vi "Navigation_start_cases_florida_rev3_joystick_cleaned.vi"() -> ()   [LabVIEW 2015]
uses:
  <vilib>/myRIO/Instrument Drivers/Onboard IO/PWM/typedefs/PWM Reference.ctl
  <vilib>/myRIO/Common/Instrument Driver Framework/Utilities/typedefs/myRIO Generic Hardware Reference.ctl
  <vilib>/myRIO/Common/Instrument Driver Framework/Utilities/typedefs/Hardware Version Enum.ctl
  <vilib>/myRIO/Common/Instrument Driver Framework/Utilities/typedefs/myRIO v1.0 Reference.ctl
  <vilib>/myRIO/Common/Instrument Driver Framework/Utilities/typedefs/Generic FPGA Reference.ctl
  <vilib>/myRIO/Common/Instrument Driver Framework/myRIO v1.0/PWM/typedefs/PWM Channels Enum.ctl
  <vilib>/myRIO/Instrument Drivers/Onboard IO/PWM/typedefs/PWM Configuration.ctl
  <vilib>/userdefined/High Color/nirio_resource_hc.ctl
  <vilib>/myRIO/Common/Instrument Driver Framework/myRIO v1.0/PWM/vis/myRIO v1.1 Open PWM.vi
  <vilib>/myRIO/Common/Instrument Driver Framework/Utilities/vis/Validate Channels.vi
  <vilib>/myRIO/Common/Instrument Driver Framework/myRIO v1.0/PWM/vis/myRIO v1.0 Reserve PWM.vi
  <vilib>/myRIO/Common/Instrument Driver Framework/myRIO v1.0/PWM/vis/myRIO v1.0 Build MUX Configuration PWM.vi
  <vilib>/myRIO/Common/Instrument Driver Framework/myRIO v1.0/Resource Manager/vis/myRIO v1.0 Reserve Channel List.vi
  <vilib>/myRIO/Common/Instrument Driver Framework/myRIO v1.0/Resource Manager/vis/myRIO v1.0 Create Configuration List.vi
  <vilib>/myRIO/Common/Instrument Driver Framework/myRIO v1.0/Resource Manager/vis/myRIO v1.0 Reserve Channel.vi
  <vilib>/myRIO/Common/Instrument Driver Framework/myRIO v1.0/Resource Manager/vis/myRIO v1.0 Unreserve Channel.vi
  <vilib>/myRIO/Common/Instrument Driver Framework/myRIO v1.0/Resource Manager/vis/myRIO v1.0 Build Mutex Name.vi
  <vilib>/FPGAPlugInAG/myRIO-1900/niLvFpga_Open_myRIO-1900.vi
  <vilib>/rvi/interface/common/dynamic/niFpgaDynamicAddResources.vi
  <vilib>/myRIO/Common/Instrument Driver Framework/Utilities/vis/FPGA Ref Manager.vi
  <vilib>/Utility/error.llb/Error Cluster From Error Code.vi
  <vilib>/myRIO/Common/Instrument Driver Framework/Utilities/vis/Ref Counter.vi
  <vilib>/rvi/errors/niLvFpgaAdjustHostInterfaceError.vi
  <vilib>/Utility/VariantDataType/GetNumericInfo.vi
  <vilib>/myRIO/Common/Instrument Driver Framework/myRIO v1.0/myRIO v1.1 Open.vi
  <vilib>/myRIO/Common/Instrument Driver Framework/Utilities/vis/IO Manager.vi
  <vilib>/myRIO/Common/Instrument Driver Framework/Utilities/vis/Configuration Manager.vi
  <vilib>/myRIO/Common/Instrument Driver Framework/myRIO v1.0/Resource Manager/vis/myRIO v1.0 Configure IO.vi
  <vilib>/myRIO/Common/Instrument Driver Framework/myRIO v1.0/myRIO v1.0 Close.vi
  <vilib>/myRIO/Common/Instrument Driver Framework/myRIO v1.0/PWM/vis/myRIO v1.0 Write PWM.vi
  <vilib>/addons/control/pid/pid.llb/PID (DBL).vi
  <vilib>/rvi/interface/nirviOpenFPGA/nirviOpenFPGA.xnode
  FPGA Bitfiles/NavigationProjec_FPGATarget2_FPGAMainNavigati_PWPHW8gwDxI.lvbitx
  <vilib>/rvi/interface/nirviReadWriteControl/nirviReadWriteControl.xnode
  <vilib>/myRIO/Instrument Drivers/Onboard IO/PWM/vis/myRIO PWM Open.xnode
  <vilib>/myRIO/Instrument Drivers/Onboard IO/PWM/PWM.lvlib
  <vilib>/myRIO/Instrument Drivers/Utilities/Utilities.lvlib
  NiFpgaLv.dll
  <vilib>/rvi/interface/Simulation/niFpgaSimulationCallBeginRW.vi
  <vilib>/addons/control/pid/NI_PID_pid.lvlib
panel:
  in  "left setpoint 7":dbl=0.06
  in  "right setpoint 7":dbl=0.06
  in  "left setpoint 6":dbl=0.06
  in  "right setpoint 6":dbl=0.06
  in  "right setpoint 5":dbl=0.1
  in  "left setpoint 5":dbl=0.06 format="%#_13g"
  in  "right setpoint 4":dbl=0.06
  in  "left setpoint 4":dbl=0.1
  in  "left setpoint 3":dbl=0.05
  in  "right setpoint 3":dbl=0.1
  in  "left setpoint 2":dbl=0.08 format="%#_13g"
  in  "right setpoint 2":dbl=0.05
  in  "y goal lower limit return":dbl=1.5
  in  "y goal upper limit return":dbl=3.5
  in  "y goal upper limit mine":dbl=9.0
  in  "y goal lower limit mine":dbl=5.0
  in  "dump y":dbl=2.5 format="%#_13g"
  out "angle goal":dbl
  out "y goal":dbl
  in  "dump x":dbl=2.0
  in  "timer control":u32=750
  in  "dumping complete":bool
  in  "digging complete?":bool
  out "start condition":dbl format="%#_13g"
  out "xstart_return":dbl
  out "start x 2":dbl=1.0
  out "goal reached 2":bool=TRUE
  out "percent away from x goal 2":dbl
  in  "x goal":dbl=9.0
  out "goal reached":bool=TRUE
  out "percent away from x goal":dbl
  in  "t backward 6":u32=3000
  in  "Tab Control":enum32{"start a", "start b"}(tab)
  in  "?":T1(tab)=enum."back arc 4 4"
  in  "right 0":dbl=-0.05
  in  "left 0":dbl=-0.05
  in  "t backward 7":u32=3000
  in  "left 1":dbl=0.1
  in  "right 1":dbl=0.05
  in  "right 2":dbl=0.05
  in  "left 2":dbl=0.1
  in  "t backward":u32=3000
  in  "t forward":u32=750
  in  "t forward once":u32=3000
  in  "right once":dbl=0.05
  in  "left once":dbl=0.1
  in  "left 7":dbl=0.1
  in  "right 7":dbl=0.05
  in  "t forward 2":u32=750
  in  "left 6":dbl=0.1
  in  "right 6":dbl=0.05
  in  "t backward 2":u32=3000
  in  "left once 2":dbl=0.1
  in  "right once 2":dbl=0.05
  in  "t forward once 2":u32=3000
  in  "left 12":dbl=0.1
  in  "right 12":dbl=0.05
  in  "left 11":dbl=0.1
  in  "right 11":dbl=0.05
  in  "left 10":dbl=0.1
  in  "right 10":dbl=0.05
  in  "forward":u32=5000
  in  "timeforward":u32=750
  in  "timeback":u32=750
  in  "Tab Control 3":T2(tab)
  in  "left 15":dbl=-0.05
  in  "right 15":dbl=-0.05
  in  "t backward 8":u32=3000
  in  "left 5":dbl=0.1
  in  "right 5":dbl=0.05
  in  "left 4":dbl=0.1
  in  "right 4":dbl=0.05
  in  "left 3":dbl=0.1
  in  "right 3":dbl=0.05
  in  "forward 6":u32=750
  in  "backward 6":u32=750
  in  "onetime 6":u32=5000
  in  "t forward once 5":u32=3000
  in  "right once 5":dbl=0.05
  in  "left once 5":dbl=0.1
  in  "left 16":dbl=0.1
  in  "right 16":dbl=0.05
  in  "t backward 5":u32=3000
  in  "left 17":dbl=0.1
  in  "right 17":dbl=0.05
  in  "t forward 5":u32=750
  in  "start condition":dbl=8.0
  out "big red button":i16
  out "y1ahead":dbl=0.09107784569025501
  out "angle error":dbl=1.4898186625859124
  out "y desired":dbl=-7.9788842668421
  out "slope desired":dbl=12.322079916445226
  out "orientation theta desired":dbl=1.4898186625859124
  out "current angle":dbl
  out "current y":dbl
  out "current x":dbl
  out "mining angle":dbl
  out "mining y":dbl
  out "mining x":dbl
  out "mining location":dbl=-1.0
  out "distance to goal":dbl=-5.348200626633382
  out "loc_y":dbl=1.4807790517807007
  out "loc_x":dbl=3.651799373366618
  out "loc_theta":dbl
  in  "motor killswitch":bool
  in  "state":dbl
  in  "Encoder Reset":bool
  out "scale":dbl
  out "reset x y 2":dbl=1.0
  out "stop motors":dbl
  out "encoder stop switch":dbl=1.0
  out "left wheels actual pwm":dbl=0.5
  out "right wheels actual pwm":dbl=0.5
  out "desired pwm right":dbl=0.5
  out "desired pwm left":dbl=0.5
  out "left setpoint":dbl
  out "right setpoint":dbl
  in  "PID Settings":enum32{"Right PID PWM", "Left PID PWM"}(tab)
  in  "output range right":cluster{"output high":dbl, "output low":dbl}={"output high"=0.15, "output low"=-0.15} {"output low" format="%.6f"; "output high" format="%.5f"}
  in  "PID gains right":T3={"proportional gain (Kc)"=0.002, "integral time (Ti, min)"=7e-07, "derivative time (Td, min)"=0.0} {"derivative time (Td, min)" format="%.8f"; "integral time (Ti, min)" format="%.8f"; "proportional gain (Kc)" format="%.8f"}
  out "dt out (s) right":dbl=0.003000000142492354 format="%.3f"
  out "PID feedback Right":dbl
  out "Elapsed Time (s) Right":dbl=3.140906810760498 caption="Elapsed Time (s)"
  in  "pid reset right":bool
  in  "output range left":cluster{"output high":dbl, "output low":dbl}={"output high"=0.15, "output low"=-0.15} {"output low" format="%.6f"; "output high" format="%.5f"}
  in  "PID gains left":T3={"proportional gain (Kc)"=0.002, "integral time (Ti, min)"=7e-07, "derivative time (Td, min)"=0.0} {"derivative time (Td, min)" format="%.8f"; "integral time (Ti, min)" format="%.8f"; "proportional gain (Kc)" format="%.8f"}
  out "dt out (s) left":dbl=0.003000000142492354 format="%.3f"
  out "PID feedback Left":dbl
  out "Elapsed Time (s) Left":dbl=3.15102481842041 caption="Elapsed Time (s)"
  in  "pid reset left":bool
  out "start angle":dbl
  out "start x":dbl=3.5057763724032824
  out "start y":dbl=1.4807790517807007
  in  "stuff that i dont want to mess with right now":T4(tab)
  out "RM Linear Velocity (rot/s)":dbl
  out "RR Rot Velocity (rot/s)":dbl
  out "LR Rot Velocity (rot/s)":dbl
  out "LM Rot Velocity (rot/s)":dbl
  out "LF Rot Velocity (rot/s)":dbl
  out "RF Linear Velocity (rot/s)":dbl
  out "Tick Count(mSec) 2":u32=223952 caption="Tick Count(mSec)"
  out "y traveled 2":dbl
  out "x traveled 2":dbl
  out "y position 2":dbl=1.4807790517807007
  out "x position 2":dbl=3.5057763724032824
  out "y dot 2":dbl
  out "distance traveled 2":dbl
  out "psi dot 2":dbl
  out "x dot 2":dbl
  out ".not. x? 2":bool
  out ".not. x? 3":bool
  out "avg ENC.B":dbl
  out "avg ENC.A":dbl
  out "ENC.B_c.CNTR":i32
  out "ENC.B_b.CNTR":i32
  out "ENC.B_a.CNTR":i32
  out "ENC.A_c.CNTR":i32
  out "ENC.A_b.CNTR":i32
  out "ENC.A_a.CNTR":i32
  out "stage set point parameters":T5(tab)=enum."mining location -1"
  in  "x straight 1 end":dbl=2.0
  in  "ypstart straight 1":dbl
  in  "ystart":dbl=1.0
  in  "yend straight 1":dbl=2.0
  in  "ypend straight 1":dbl
  out "a":dbl=1.7573967372023482
  out "b":dbl=-14.513750148940964
  out "c":dbl=36.96623974933568
  out "d":dbl=-23.9366528005263
  out "x turn end":dbl=7.0
  out "x straight 2 end":dbl=10.0
  in  "mining y 1":dbl=2.0
  in  "mining angle 1":dbl
  in  "mining x 1":dbl=20.0
  in  "mining angle -1":dbl
  in  "mining y -1":dbl=7.0
  in  "mining x -1":dbl=20.0
  # "go up in y"
  # "go down in y"
  # "go straight"
  # "Position Information"
  # "straight arc back straight arc arc"
  # "move cases along"
  # "end state 0\ngo to state 1"
  # "end state 1\ngo to state 2"
  # "end state 2\ngo to state 3"
  # "end state 3\ngo to state 4"
  # "end state 4\ngo to state 0"
  # "same thing, redundant \nbut can be changed to \nsomething useful later"
  # "this must be true to \ninitialize the routine"
  # "go through the 3\n movement cases"
  # "go through the 3\n movement cases"
  # "same as the start a arc arc"
  # "Stop Flags \n1=go \n0=stop"
  # "PWM Setpoint"
  # "Initial condtions"
  # "Encoder Values"
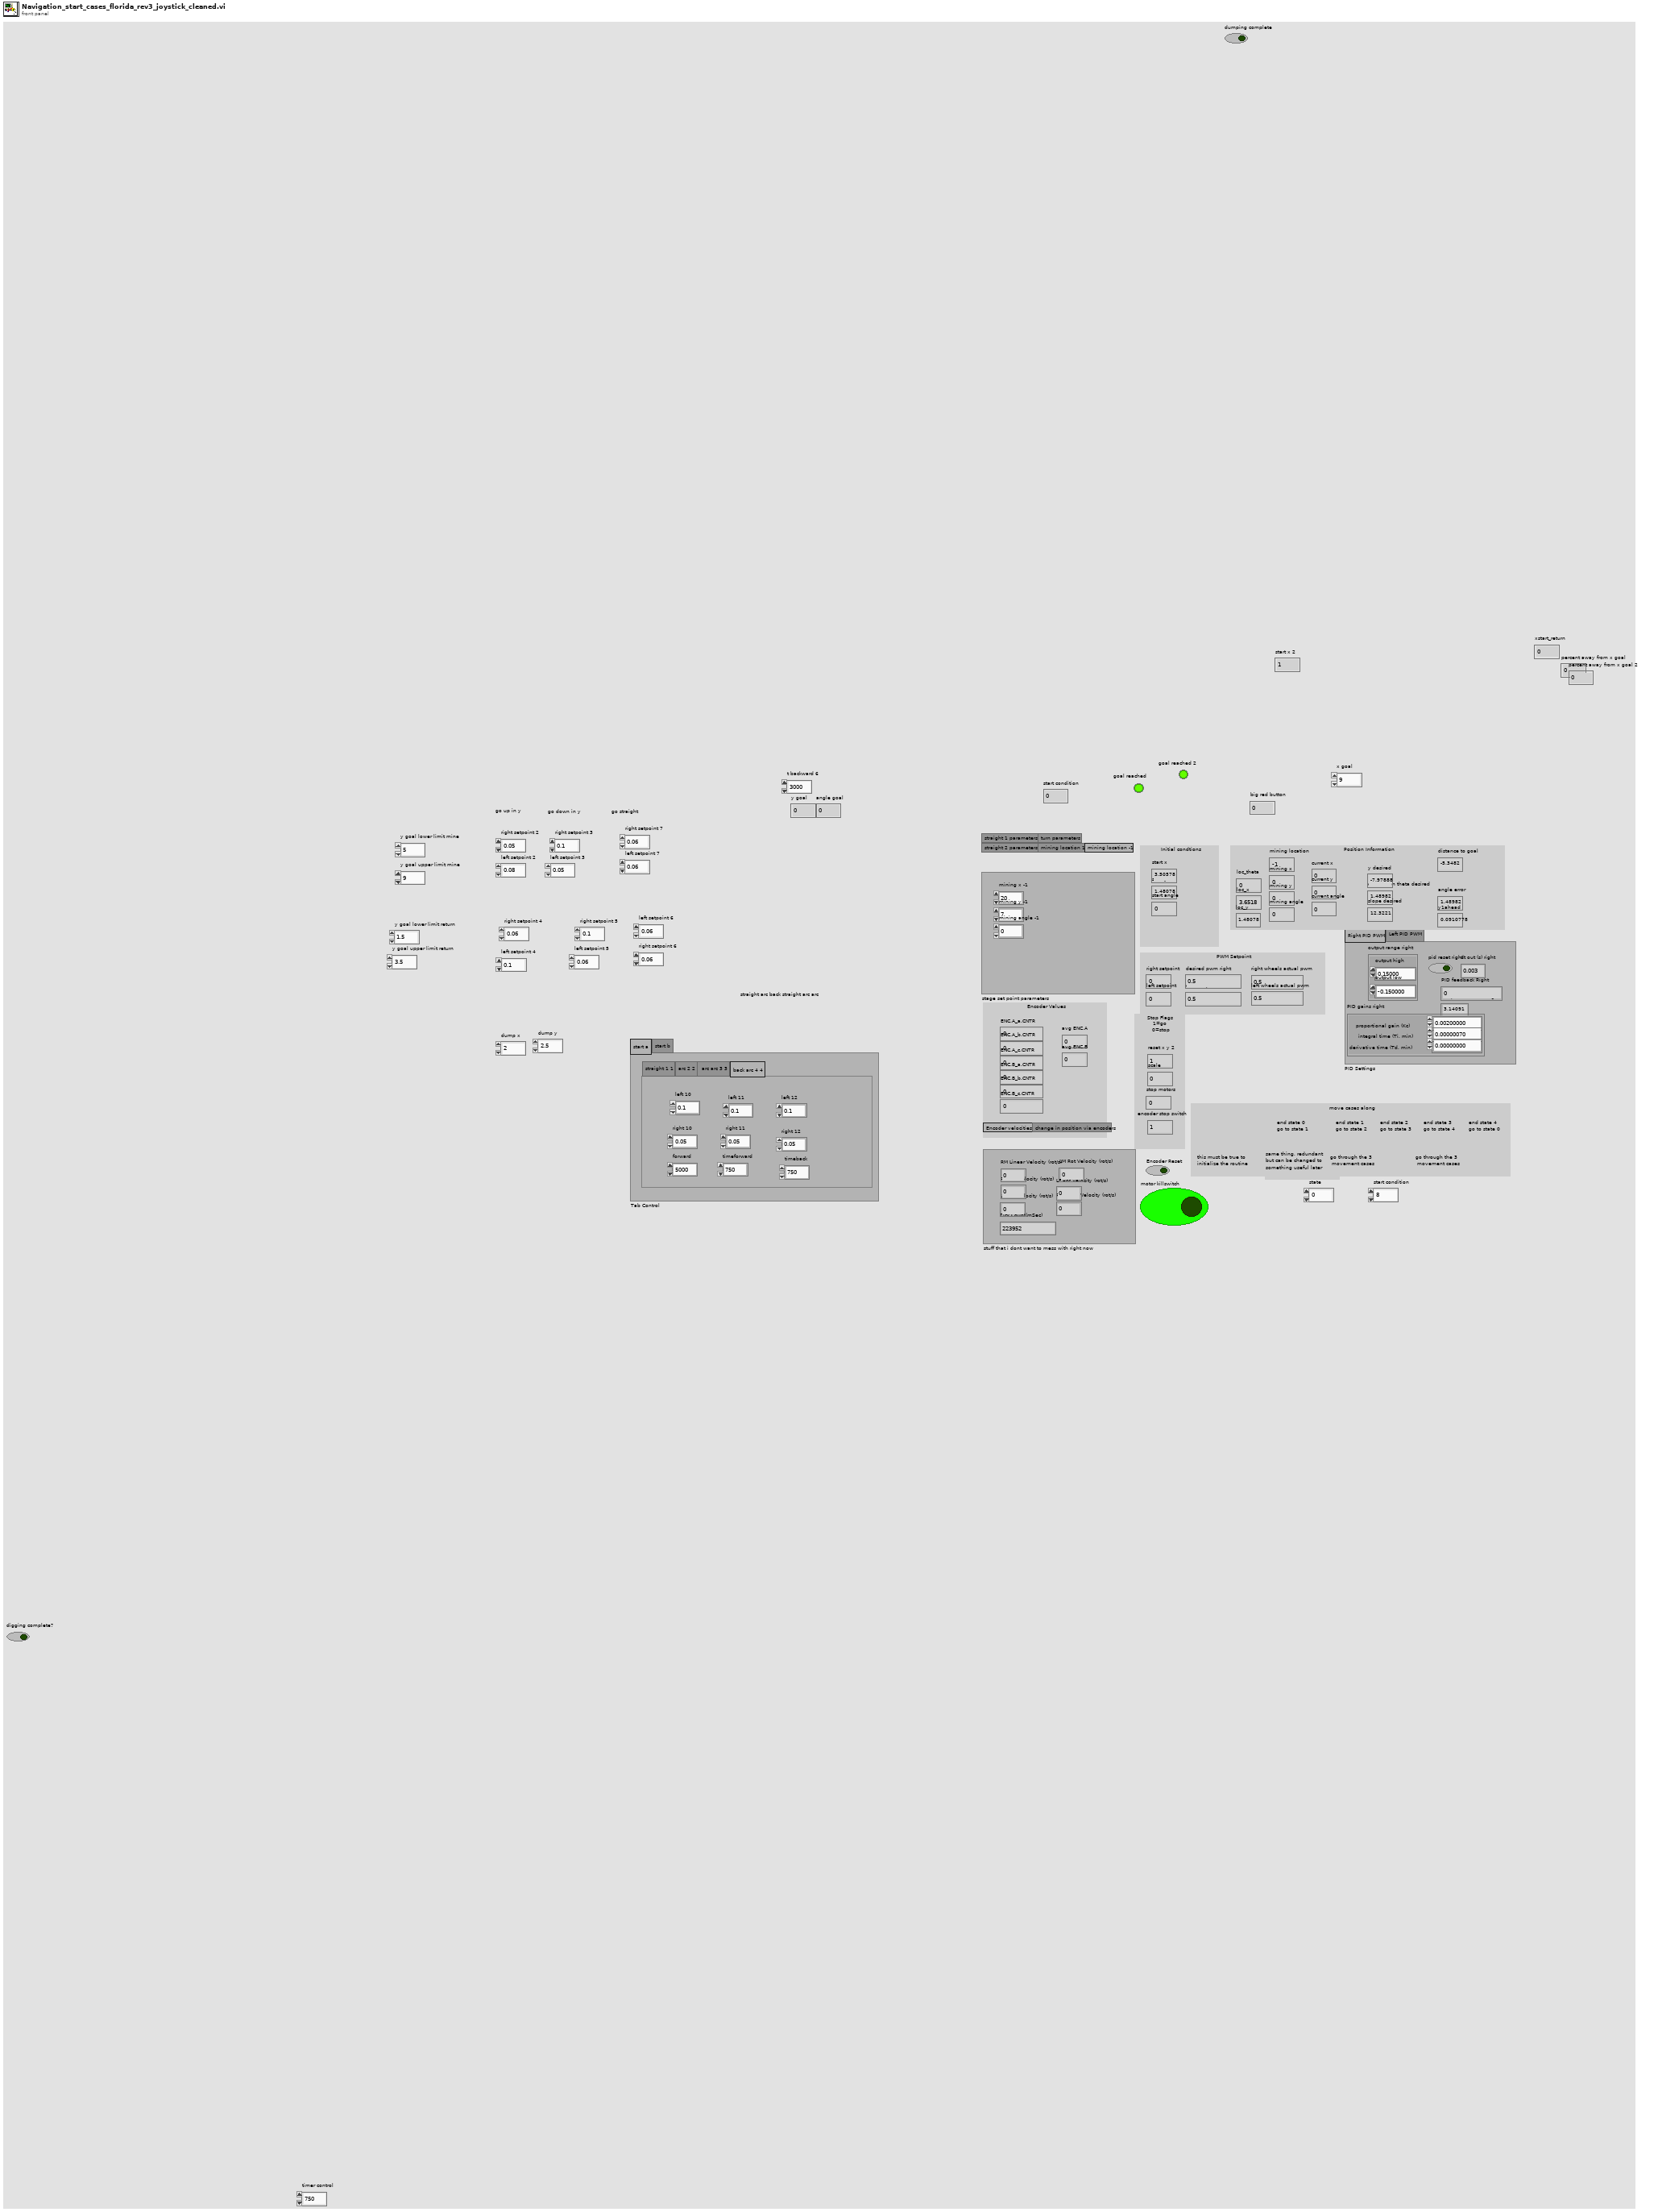
[diagram p1: front panel]
types:
  T1 = enum32{"straight 1 1", "arc 2 2", "arc arc 3 3 ", "back arc 4 4"}
  T2 = enum32{"straight 1 5", "arc 2 6", "arc arc 3", "back arc 4 7"}
  T3 = cluster{"proportional gain (Kc)":dbl, "integral time (Ti, min)":dbl, "derivative time (Td, min)":dbl}
  T4 = enum32{"Encoder velocities", "change in position via encoders"}
  T5 = enum32{"straight 1 parameters", "turn parameters", "straight 2 parameters", "mining location 1", "mining location -1"}
  T6 = typedef "nirio_resource_hc.ctl" = tag
  T7 = typedef "Hardware Version Enum.ctl" = enum16{"Unknown", "myRIO-1900", "myRIO-1950", "roboRIO"}
  T8 = typedef "PWM.lvlib/PWM Reference.ctl" = cluster{"myRIO Reference":T9, "PWM Channels Enum":T12, "PWM Configuration":T13}
  T9 = typedef "myRIO Generic Hardware Reference.ctl" = cluster{"myRIO Model":T7, "myRIO Hardware Reference":T10}
  T10 = typedef "myRIO v1.0 Reference.ctl" = cluster{"Generic FPGA Reference":T11, "Allow multiple opens":bool}
  T11 = typedef "Generic FPGA Reference.ctl" = refnum<k20>
  T12 = typedef "PWM Channels Enum.ctl" = enum16{"Not Connected", "C/PWM0", "C/PWM1", "A/PWM0", "A/PWM1", "A/PWM2", "B/PWM0", "B/PWM1", "B/PWM2", "PWM/PWM0", "PWM/PWM1", "PWM/PWM2", "PWM/PWM3", "PWM/PWM4", "PWM/PWM5", "PWM/PWM6", "PWM/PWM7", "PWM/PWM8", "PWM/PWM9"}
  T13 = typedef "PWM.lvlib/PWM Configuration.ctl" = cluster{"Frequency":dbl, "Duty Cycle":dbl}
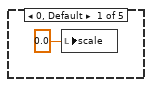
[diagram p3: hidden frame]
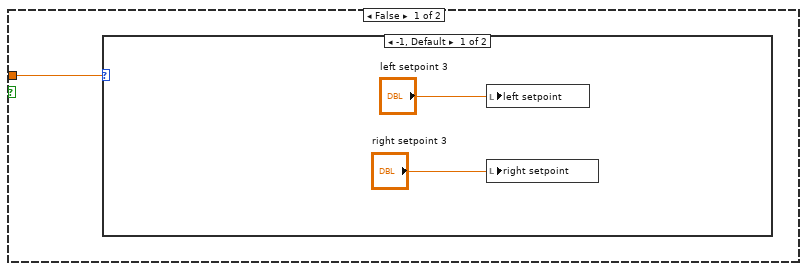
[diagram p4: hidden frame]
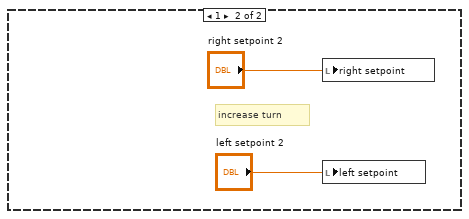
[diagram p5: hidden frame]
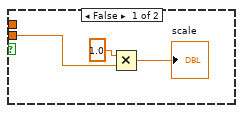
[diagram p6: hidden frame]
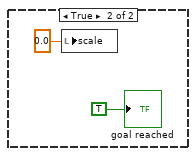
[diagram p7: hidden frame]
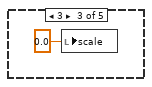
[diagram p8: hidden frame]
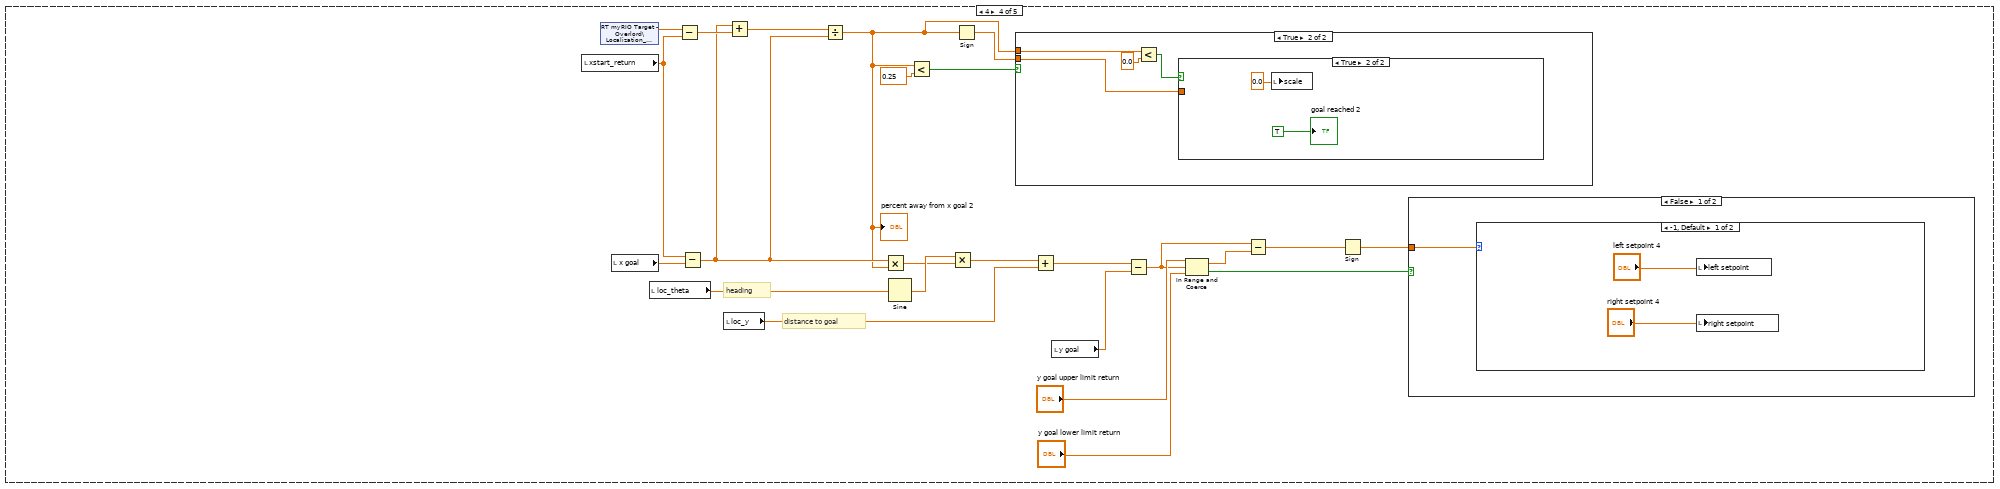
[diagram p9: hidden frame]
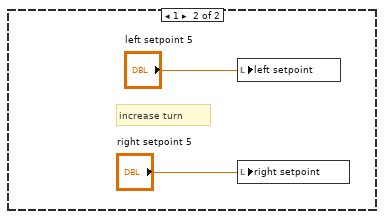
[diagram p10: hidden frame]
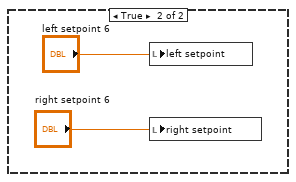
[diagram p11: hidden frame]
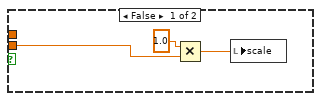
[diagram p12: hidden frame]
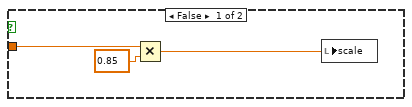
[diagram p13: hidden frame]
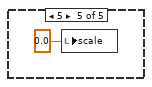
[diagram p14: hidden frame]
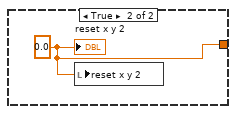
[diagram p15: hidden frame]
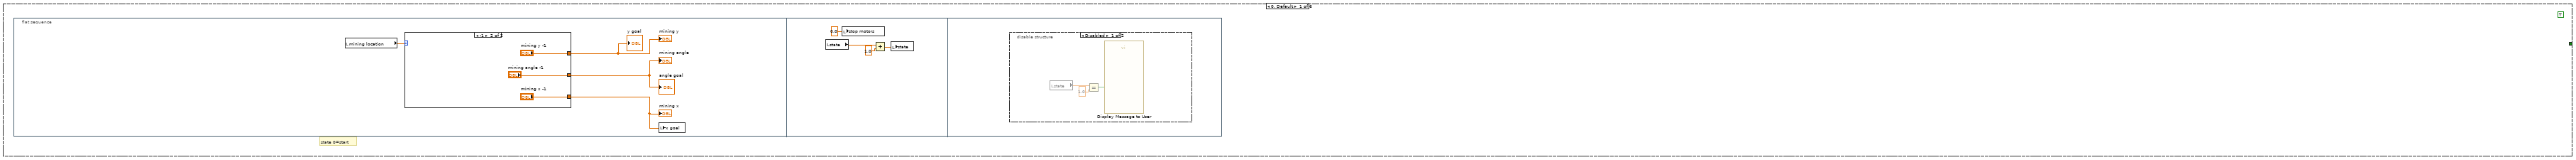
[diagram p16: hidden frame]
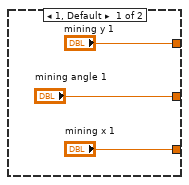
[diagram p17: hidden frame]
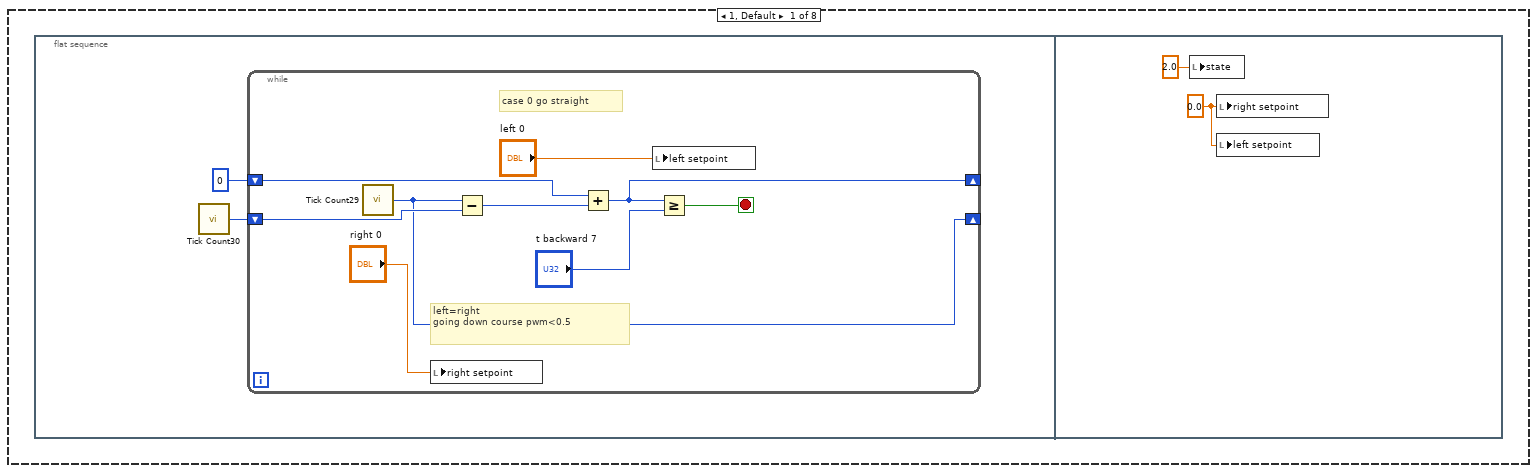
[diagram p19: hidden frame]
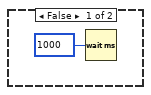
[diagram p20: hidden frame]
diagram:
  n1 = flat-sequence {
    tunnel: [w35] -> w32
    tunnel: [w35] -> w31
    tunnel: [w48] -> w20
    tunnel: [w59] -> w18
    tunnel: [w55] -> w16
    tunnel: [w54] -> w14
    tunnel: [w53] -> w12
    tunnel: [w52] -> w10
    tunnel: [w51] -> w8
    tunnel: [w50] -> w6
    tunnel: w32 -> [w49]
    tunnel: [w49] -> w4
    tunnel: w31 -> [w50]
    tunnel: [w48] -> w2
    tunnel: w20 -> [w181]
    tunnel: [w181] -> w19
    tunnel: w18 -> [w180]
    tunnel: [w180] -> w17
    tunnel: w16 -> [w179]
    tunnel: [w179] -> w15
    tunnel: w14 -> [w178]
    tunnel: [w178] -> w13
    tunnel: w12 -> [w177]
    tunnel: [w177] -> w11
    tunnel: w10 -> [w176]
    tunnel: [w176] -> w9
    tunnel: w8 -> [w175]
    tunnel: [w175] -> w7
    tunnel: w6 -> [w174]
    tunnel: [w174] -> w5
    tunnel: w4 -> [w173]
    tunnel: [w173] -> w3
    tunnel: w2 -> [w172]
    tunnel: [w172] -> w1
    tunnel: w19 -> [w192]
    tunnel: [w192] -> w30
    tunnel: w17 -> [w191]
    tunnel: [w191] -> w29
    tunnel: w15 -> [w190]
    tunnel: [w190] -> w28
    tunnel: w13 -> [w189]
    tunnel: [w189] -> w27
    tunnel: w11 -> [w188]
    tunnel: [w188] -> w26
    tunnel: w9 -> [w187]
    tunnel: [w187] -> w25
    tunnel: w7 -> [w186]
    tunnel: [w186] -> w24
    tunnel: w5 -> [w185]
    tunnel: [w185] -> w23
    tunnel: w3 -> [w184]
    tunnel: [w184] -> w22
    tunnel: w1 -> [w183]
    tunnel: [w183] -> w21
    tunnel: w30 -> [_]
    tunnel: w29 -> [w206]
    tunnel: w28 -> [w212]
    tunnel: w27 -> [w209]
    tunnel: w26 -> [w208]
    tunnel: w25 -> [w207]
    tunnel: w24 -> [w211]
    tunnel: w23 -> [w214]
    tunnel: w22 -> [w213]
    tunnel: w21 -> [w210]
    frame #0 {
      n2 = xnode "Open FPGA VI Reference"("resource name"=tag "RIO0") -> ("FPGA VI Reference Out"=w34:refnum<k20>)  [unwired: 1 in, 1 out]
      n3 = call <vilib>:"Set Custom Bitfile.vi"("Custom FPGA Reference In"=w34) -> ("Custom FPGA Reference Out"=w36:refnum<k20>)  [unwired: 9 in, 1 out]
      n4 = flat-sequence {
        tunnel: w36 -> [w41]
        tunnel: [w39] -> w38
        tunnel: w38 -> [w43]
        tunnel: [w43] -> w37
        tunnel: w37 -> [w46]
        tunnel: [w45] -> w35
        frame #0 {
          w40 = u8 32 ("SYS.SELECTA")
          w42 = u8 3 ("ENC.B_c.CNFG")
          n5 = xnode "Read/Write Control"("FPGA VI Reference In"=w41, "ENC.A_a.CNFG"=w42, "ENC.A_b.CNFG"=w42, "ENC.A_c.CNFG"=w42, "ENC.B_a.CNFG"=w42, "ENC.B_b.CNFG"=w42, "ENC.B_c.CNFG"=w42, "SYS.SELECTA"=w40, "SYS.SELECTB"=w40) -> ("FPGA VI Reference Out"=w39:refnum<k20>)  [unwired: 1 in, 1 out]
        }
        frame #1 {
          n6 = Wait (ms)(milliseconds to wait=u32 10) -> ()  [unwired: 1 out]
        }
        frame #2 {
          w47 = u8 1 ("ENC.B_c.CNFG")
          n7 = xnode "Read/Write Control"("FPGA VI Reference In"=w46, "ENC.A_a.CNFG"=w47, "ENC.A_b.CNFG"=w47, "ENC.A_c.CNFG"=w47, "ENC.B_a.CNFG"=w47, "ENC.B_b.CNFG"=w47, "ENC.B_c.CNFG"=w47) -> ("FPGA VI Reference Out"=w45:refnum<k20>)  [unwired: 1 in, 1 out]
        }
      }
    }
    frame #1 {
      w56 = 0.5 ("Duty Cycle")
      w48 = 333.333 ("Frequency [Hz]")
      w70 = tag "B/PWM2"  # Right rear ch
      w71 = tag "B/PWM0"  # Right mid ch
      w72 = tag "B/PWM1"  # Right front ch
      w73 = tag "A/PWM2"  # Left rear ch
      w74 = tag "A/PWM1"  # Left mid ch
      w75 = tag "A/PWM0"  # Left front ch
      n8 = xnode "Left Front"("Channel Name"=w75) -> ("PWM Ref Out"=w69:T8)  [unwired: 2 in, 1 out]
      n9 = xnode "Left Rear"("Channel Name"=w73) -> ("PWM Ref Out"=w67:T8)  [unwired: 2 in, 1 out]
      n10 = xnode "Right  Front"("Channel Name"=w72) -> ("PWM Ref Out"=w66:T8)  [unwired: 2 in, 1 out]
      n11 = xnode "Right  Rear"("Channel Name"=w70) -> ("PWM Ref Out"=w64:T8)  [unwired: 2 in, 1 out]
      n12 = xnode "Right  Mid"("Channel Name"=w71) -> ("PWM Ref Out"=w65:T8)  [unwired: 2 in, 1 out]
      n13 = xnode "Left Mid"("Channel Name"=w74) -> ("PWM Ref Out"=w68:T8)  [unwired: 2 in, 1 out]
      n14 = call <vilib>:"Set Frequency.vi"("Frequency [Hz]"=w48, "PWM Ref In"=w69) -> ("PWM Ref Out"=w63:T8)  [unwired: 7 in, 1 out]
      n15 = call <vilib>:"Set Frequency.vi"("Frequency [Hz]"=w48, "PWM Ref In"=w68) -> ("PWM Ref Out"=w57:T8)  [unwired: 7 in, 1 out]
      n16 = call <vilib>:"Set Frequency.vi"("Frequency [Hz]"=w48, "PWM Ref In"=w67) -> ("PWM Ref Out"=w58:T8)  [unwired: 7 in, 1 out]
      n17 = call <vilib>:"Set Frequency.vi"("Frequency [Hz]"=w48, "PWM Ref In"=w66) -> ("PWM Ref Out"=w60:T8)  [unwired: 7 in, 1 out]
      n18 = call <vilib>:"Set Frequency.vi"("Frequency [Hz]"=w48, "PWM Ref In"=w64) -> ("PWM Ref Out"=w62:T8)  [unwired: 7 in, 1 out]
      n19 = call <vilib>:"Set Frequency.vi"("Frequency [Hz]"=w48, "PWM Ref In"=w65) -> ("PWM Ref Out"=w61:T8)  [unwired: 7 in, 1 out]
      n20 = call <vilib>:"Set Duty Cycle.vi"("Duty Cycle"=w56, "PWM Ref In"=w63) -> ("PWM Ref Out"=w51:T8)  [unwired: 7 in, 1 out]
      n21 = call <vilib>:"Set Duty Cycle.vi"("Duty Cycle"=w56, "PWM Ref In"=w57) -> ("PWM Ref Out"=w52:T8)  [unwired: 7 in, 1 out]
      n22 = call <vilib>:"Set Duty Cycle.vi"("Duty Cycle"=w56, "PWM Ref In"=w58) -> ("PWM Ref Out"=w59:T8)  [unwired: 7 in, 1 out]
      n23 = call <vilib>:"Set Duty Cycle.vi"("Duty Cycle"=w56, "PWM Ref In"=w60) -> ("PWM Ref Out"=w55:T8)  [unwired: 7 in, 1 out]
      n24 = call <vilib>:"Set Duty Cycle.vi"("Duty Cycle"=w56, "PWM Ref In"=w62) -> ("PWM Ref Out"=w53:T8)  [unwired: 7 in, 1 out]
      n25 = call <vilib>:"Set Duty Cycle.vi"("Duty Cycle"=w56, "PWM Ref In"=w61) -> ("PWM Ref Out"=w54:T8)  [unwired: 7 in, 1 out]
    }
    frame #2 {
      n26 = while {
        stop <- w182 stop-if-true
        n27 = shared-variable "RT myRIO Target - Navigation\\Joystick_Variables.lvlib\\Start Run"() -> (w182:bool)  [unwired: 1 in, 1 out]
      }
    }
    frame #3 {
      n28 = while {
        stop <- w197 stop-if-true
        n29 = shared-variable "RT myRIO Target - Navigation\\Joystick_Variables.lvlib\\Auto_Manual"() -> (w196:bool)  [unwired: 1 in, 1 out]
        n30 = shared-variable "RT myRIO Target - Overlord\\Localization_Variables_r0.lvlib\\Position_Lock"() -> (w195:bool)  [unwired: 1 in, 1 out]
        n31 = Not(x=w196) -> (.not. x?=w193:bool)
        n32 = Or(x=w195, y=w193) -> (x .or. y?=w194:bool)
        n33 = case shown="True" w194 {
          selector: w194 -> [_ w203]
          tunnel: [_ w203] -> w197
          frame False {
          }
          frame True {
            n34 = shared-variable "RT myRIO Target - Overlord\\Localization_Variables_r0.lvlib\\loc_x"() -> (→"start x":dbl)  [unwired: 1 in, 1 out]
            n35 = shared-variable "RT myRIO Target - Overlord\\Localization_Variables_r0.lvlib\\loc_y"() -> (→"start y":dbl)  [unwired: 1 in, 1 out]
            n36 = shared-variable "RT myRIO Target - Overlord\\Localization_Variables_r0.lvlib\\loc_theta"() -> (→"start angle":dbl)  [unwired: 1 in, 1 out]
            n37 = Wait (ms)(milliseconds to wait=u32 500) -> ()  [unwired: 1 out]
            "stop motors" <- 0.0 ("stop motors")
          }
        }
      }
    }
    frame #4 {
      (unwired) FALSE
      # "Uses quadrature encoder tick count to calculate rotational and linear velocity for a wheel."
      # "20ms loop delay to allow the encoder to travel far enough for a good update. 20ms provides 50Hz update rate to match motor PWM output rate."
      n38 = flat-sequence {
        frame #0 {
          # "this calculates from the \nmeasured start to the desired end"
          n39 = local read "x straight 1 end"() -> (w333:dbl)
          n40 = local read "start x"() -> (w334:dbl)
          n41 = call "path coefs.vi"("ypend"="ypend straight 1", "ypstart"="ypstart straight 1", "yend"="yend straight 1", "ystart"="ystart", "xend"=w333, "xstart"=w334) -> ("d"=→"d":dbl, "c"=→"c":dbl, "b"=→"b":dbl, "a"=→"a":dbl)  [unwired: 2 in]
        }
      }
      n42 = call "Tick Count28"() -> ("Tick Count(mSec)"=w205:u32)
      n43 = while {
        stop <- FALSE stop-if-true
        n44 = shared-variable "RT myRIO Target - Overlord\\Localization_Variables_r0.lvlib\\loc_y"() -> (→"loc_y":dbl)  [unwired: 1 in, 1 out]
        n45 = shared-variable "RT myRIO Target - Overlord\\Localization_Variables_r0.lvlib\\loc_x"() -> (w769:dbl)  [unwired: 1 in, 1 out]
        "loc_x" <- w769
        n46 = shared-variable "RT myRIO Target - Overlord\\Localization_Variables_r0.lvlib\\loc_theta"() -> (→"loc_theta":dbl)  [unwired: 1 in, 1 out]
        n47 = local read "x goal"() -> (w768:dbl)
        n48 = Subtract(x=w769, y=w768) -> (x-y=→"distance to goal":dbl)
      }
      n49 = while {
        stop <- FALSE stop-if-true
        n50 = local read "current x"() -> (w327:dbl)
        n51 = local read "a"() -> (w331:dbl)
        n52 = local read "b"() -> (w330:dbl)
        n53 = local read "c"() -> (w329:dbl)
        n54 = local read "d"() -> (w328:dbl)
        n55 = formula code="yshould=(a*x**3)/3+(b*x**2)/3+(c*x)/3+d/3;\ny1ahead=(a*(x+1)**3)/3+(b*(x+1)**2)/3+(c*(x+1))/3+d/3;\nslope=(a*x**2 + (2*b*x)/3 + c/3);\nrobot_orientation_theta=(atan(slope));\nleftwheel_x=(-1*sin(robot_orientation_theta)+x);\nrightwheel_x=(1*sin(robot_orientation_theta)+x);\nleftwheel_y=(1*cos(robot_orientation_theta)+yshould);\nrightwheel_y=(-1*cos(robot_orientation_theta)+yshould);"("a"=w331, "b"=w330, "c"=w329, "d"=w328, "x"=w327) -> ("yshould"=→"y desired":dbl, "slope"=→"slope desired":dbl, "robot_orientation_theta"=w324:dbl, "y1ahead"=→"y1ahead":dbl)  [unwired: 4 out]
        "orientation theta desired" <- w324
        n56 = local read "current angle"() -> (w323:dbl)
        n57 = Subtract(x=w324, y=w323) -> (x-y=→"angle error":dbl)
      }
      n58 = while {
        shift-right: [w832] -> _
        shift-left: _ -> [w870]
        shift-right: [w829] -> _
        shift-left: _ -> [w869]
        shift-right: [w831] -> _
        shift-left: _ -> [w844]
        shift-right: [w830] -> _
        shift-left: _ -> [w843]
        stop <- FALSE stop-if-true
        w865 = 28.0  # width wheel to wheel
        w866 = 4.0  # wheel radius
        n59 = local read "reset x y 2"() -> (w828:dbl)
        n60 = call "Wait3"("Count(mSec)"=u32 20) -> ("Tick Count(mSec)"=→"Tick Count(mSec) 2":u32)
        n61 = Multiply(x=w828, y=w844) -> (x*y=w835:dbl)
        n62 = Multiply(x=w828, y=w870) -> (x*y=w836:dbl)
        n63 = Multiply(x=w828, y=w869) -> (x*y=w833:dbl)
        n64 = Multiply(x=w828, y=w843) -> (x*y=w834:dbl)
        n65 = local read "ENC.A_a.CNTR"() -> (w878:i32)
        n66 = local read "ENC.A_b.CNTR"() -> (w877:i32)
        n67 = local read "ENC.B_b.CNTR"() -> (w874:i32)
        n68 = local read "ENC.A_c.CNTR"() -> (w876:i32)
        n69 = local read "ENC.B_a.CNTR"() -> (w875:i32)
        n70 = local read "ENC.B_c.CNTR"() -> (w873:i32)
        n71 = Compound Arithmetic op=ADD(w878, w877, w876) -> (w882:i32)
        n72 = Compound Arithmetic op=ADD(w875, w874, w873) -> (w881:i32)
        n73 = Divide(x=w882, y=2) -> (x/y=w871:dbl)
        "avg ENC.A" <- w871
        n74 = Divide(x=w881, y=3) -> (x/y=w868:dbl)
        "avg ENC.B" <- w868
        n75 = Subtract(x=w871, y=w836) -> (x-y=w859:dbl)
        n76 = Subtract(x=w868, y=w833) -> (x-y=w858:dbl)
        n77 = Add(x=w859, y=w858) -> (x+y=w863:dbl)
        n78 = Divide(x=w866, y=w865) -> (x/y=w861:dbl)
        n79 = Square(x=w859) -> (x^2=w856:dbl)
        n80 = Square(x=w858) -> (x^2=w857:dbl)
        n81 = Subtract(x=w859, y=w858) -> (x-y=w862:dbl)
        n82 = Divide(x=w866, y=2.0) -> (x/y=w864:dbl)
        n83 = Add(x=w856, y=w857) -> (x+y=w855:dbl)
        n84 = Multiply(x=w863, y=w864) -> (x*y=w852:dbl)
        n85 = Multiply(x=w862, y=w861) -> (x*y=→"psi dot 2":dbl)
        n86 = Inverse Tangent(1:w862) -> (0:w860:dbl)
        n87 = Sine(x=w860) -> (sin(x)=w854:dbl)
        n88 = Cosine(x=w860) -> (cos(x)=w853:dbl)
        n89 = local read "reset x y 2"() -> (w826:dbl)
        n90 = Square Root(x=w855) -> (sqrt(x)=w849:dbl)
        n91 = Multiply(x=w852, y=w854) -> (x*y=w851:dbl)
        "y dot 2" <- w851
        n92 = Multiply(x=w852, y=w853) -> (x*y=w850:dbl)
        "x dot 2" <- w850
        n93 = Multiply(x=w871, y=w826) -> (x*y=w832:dbl)
        n94 = Multiply(x=w868, y=w826) -> (x*y=w829:dbl)
        n95 = Multiply(x=w849, y=w826) -> (x*y=w827:dbl)
        "distance traveled 2" <- w827
        n96 = Multiply(x=w827, y=w851) -> (x*y=w847:dbl)
        "y traveled 2" <- w847
        n97 = Multiply(x=w827, y=w850) -> (x*y=w848:dbl)
        "x traveled 2" <- w848
        n98 = Add(x=w835, y=w847) -> (x+y=w838:dbl)
        n99 = Add(x=w834, y=w848) -> (x+y=w846:dbl)
        n100 = Multiply(x=w826, y=w838) -> (x*y=w831:dbl)
        n101 = Multiply(x=w846, y=w826) -> (x*y=w830:dbl)
        n102 = Divide(x=w838, y=9600.0) -> (x/y=w842:dbl)
        n103 = Divide(x=w846, y=9600.0) -> (x/y=w841:dbl)
        n104 = local read "start y"() -> (w840:dbl)
        n105 = local read "start x"() -> (w839:dbl)
        n106 = Add(x=w842, y=w840) -> (x+y=→"y position 2":dbl)
        n107 = Add(x=w841, y=w839) -> (x+y=→"x position 2":dbl)
      }
      n108 = while {
        tunnel: w211 -> [w785]
        tunnel: [w815] -> _
        tunnel: w210 -> [w803]
        shift-right: [w782] -> _
        shift-left: _ -> [w811]
        shift-right: ["pid reset left"] -> _
        shift-left: _ -> [w798]
        tunnel: [w803] -> _
        tunnel: w207 -> [w805]
        tunnel: w206 -> [w804]
        stop <- "pid reset left" stop-if-true
        # "*****\n\n(true is supposed\nto be 0)"
        n109 = call "Elapsed Time2"("Reset"=w798) -> ("Elapsed Time (s)"=w797:dbl, "Time has Elapsed"=w799:bool)  [unwired: 11 in, 6 out]
        "Elapsed Time (s) Left" <- w797
        n110 = local read "scale"() -> (w790:dbl)
        n111 = Not(x=w799) -> (.not. x?=w810:bool)
        ".not. x? 3" <- w810
        n112 = Greater?(x=w790, y=0.0) -> (0:w793:bool)
        n113 = Greater Or Equal?(x=w797, y=4.0) -> (x >= y?=w795:bool)
        n114 = case shown="False" w795 {
          tunnel: [1.0 1.0] -> _
          frame False {
          }
          frame True {
          }
        }
        n115 = case shown="False" w793 {
          tunnel: [w818 w819] -> w802
          frame False {
            n116 = local read "right setpoint"() -> (w818:dbl)
          }
          frame True {
            n117 = local read "left setpoint"() -> (w819:dbl)
          }
        }
        n118 = local read "big red button"() -> (w787:i16)
        n119 = shared-variable "RT myRIO Target - Navigation\\Joystick_Variables.lvlib\\Auto_Manual"() -> (w783:bool)  [unwired: 1 in, 1 out]
        n120 = Multiply(x=w802, y=w787) -> (x*y=w788:dbl)
        n121 = local read "stop motors"() -> (w806:dbl)
        n122 = shared-variable "RT myRIO Target - Overlord\\Localization_Variables_r0.lvlib\\loc_x"() -> (w776:dbl)  [unwired: 1 in, 1 out]
        n123 = local read "encoder stop switch"() -> (w800:dbl)
        n124 = case shown="False" w783 {
          tunnel: [w816 0.0] -> w786
          frame False {
            n125 = shared-variable "RT myRIO Target - Navigation\\Joystick_Variables.lvlib\\Left Duty Cycle"() -> (w816:dbl)  [unwired: 1 in, 1 out]
          }
          frame True {
          }
        }
        n126 = Multiply(x=w790, y=w788) -> (x*y=w791:dbl)
        n127 = Multiply(x=w806, y=w791) -> (x*y=w801:dbl)
        n128 = Greater?(x=w776, y=0.5) -> (0:w775:bool)
        n129 = Add(x=0.5, y=w791) -> (x+y=→"desired pwm left":dbl)
        n130 = Multiply(x=w801, y=w800) -> (x*y=w789:dbl)
        n131 = Boolean To (0,1)(Boolean=w775) -> (0, 1=w777:i16)
        n132 = Multiply(x=w777, y=w789) -> (x*y=w778:dbl)
        n133 = call-poly <vilib>:"PID.vi"("reinitialize? (F)"=w810, "output range"="output range left", "PID gains"="PID gains left", "process variable"=w811, "setpoint"=w778) -> ("dt out (s)"=→"dt out (s) left":dbl, "output"=w782:dbl)  [unwired: 5 in]
        n134 = Boolean To (0,1)(Boolean=w783) -> (0, 1=w780:i16)
        n135 = Add(x=0.5, y=w782) -> (x+y=w781:dbl)
        n136 = Multiply(x=w781, y=w780) -> (x*y=w779:dbl)
        n137 = Add(x=w779, y=w786) -> (x+y=w784:dbl)
        "left wheels actual pwm" <- w784
        n138 = call <vilib>:"Set Duty Cycle and Frequency.vi"("Frequency [Hz]"=w803, "Duty Cycle"=w784, "PWM Ref In"=w805) -> ()  [unwired: 6 in, 2 out]
        n139 = call <vilib>:"Set Duty Cycle and Frequency.vi"("Frequency [Hz]"=w803, "Duty Cycle"=w784, "PWM Ref In"=w804) -> ()  [unwired: 6 in, 2 out]
        n140 = call <vilib>:"Set Duty Cycle and Frequency.vi"("Frequency [Hz]"=w803, "Duty Cycle"=w784, "PWM Ref In"=w785) -> ("PWM Ref Out"=w815:T8)  [unwired: 6 in, 1 out]
        "PID feedback Left" <- w811
      }
      n141 = while {
        tunnel: w212 -> [w926]
        tunnel: [w915] -> _
        shift-right: [w890] -> _
        shift-left: _ -> [w922]
        shift-right: ["pid reset right"] -> _
        shift-left: _ -> [w910]
        tunnel: w210 -> [w915]
        tunnel: w209 -> [w917]
        tunnel: w208 -> [w916]
        stop <- "pid reset right" stop-if-true
        # "******"
        n142 = local read "scale"() -> (w903:dbl)
        n143 = Greater?(x=w903, y=0.0) -> (0:w901:bool)
        n144 = case shown="False" w901 {
          tunnel: [w929 w930] -> w900
          frame False {
            n145 = local read "left setpoint"() -> (w929:dbl)
          }
          frame True {
            n146 = local read "right setpoint"() -> (w930:dbl)
          }
        }
        n147 = local read "big red button"() -> (w897:i16)
        n148 = call "Elapsed Time"("Reset"=w910) -> ("Elapsed Time (s)"=w909:dbl, "Time has Elapsed"=w907:bool)  [unwired: 11 in, 6 out]
        "Elapsed Time (s) Right" <- w909
        n149 = Multiply(x=w897, y=w900) -> (x*y=w898:dbl)
        n150 = local read "encoder stop switch"() -> (w912:dbl)
        n151 = shared-variable "RT myRIO Target - Navigation\\Joystick_Variables.lvlib\\Auto_Manual"() -> (w893:bool)  [unwired: 1 in, 1 out]
        n152 = shared-variable "RT myRIO Target - Overlord\\Localization_Variables_r0.lvlib\\loc_x"() -> (w889:dbl)  [unwired: 1 in, 1 out]
        n153 = Multiply(x=w903, y=w898) -> (x*y=w914:dbl)
        n154 = Not(x=w907) -> (.not. x?=w921:bool)
        ".not. x? 2" <- w921
        n155 = Greater Or Equal?(x=w909, y=4.0) -> (x >= y?=w906:bool)
        n156 = local read "stop motors"() -> (w904:dbl)
        n157 = case shown="False" w893 {
          tunnel: [w927 0.0] -> w896
          frame False {
            n158 = shared-variable "RT myRIO Target - Navigation\\Joystick_Variables.lvlib\\Right Duty Cycle"() -> (w927:dbl)  [unwired: 1 in, 1 out]
          }
          frame True {
          }
        }
        n159 = case shown="False" w906 {
          tunnel: [1.0 1.0] -> w911
          frame False {
          }
          frame True {
          }
        }
        n160 = Multiply(x=w914, y=w912) -> (x*y=w913:dbl)
        n161 = Add(x=0.5, y=w914) -> (x+y=→"desired pwm right":dbl)
        n162 = Greater?(x=w889, y=0.5) -> (0:w885:bool)
        n163 = Multiply(x=w904, y=w913) -> (x*y=w905:dbl)
        n164 = Boolean To (0,1)(Boolean=w885) -> (0, 1=w887:i16)
        n165 = Multiply(x=w887, y=w905) -> (x*y=w888:dbl)
        n166 = Multiply(x=w888, y=w911) -> (x*y=w884:dbl)
        n167 = call-poly <vilib>:"PID.vi"("reinitialize? (F)"=w921, "output range"="output range right", "PID gains"="PID gains right", "process variable"=w922, "setpoint"=w884) -> ("dt out (s)"=→"dt out (s) right":dbl, "output"=w890:dbl)  [unwired: 5 in]
        n168 = Boolean To (0,1)(Boolean=w893) -> (0, 1=w891:i16)
        n169 = Add(x=0.5, y=w890) -> (x+y=w895:dbl)
        n170 = Multiply(x=w895, y=w891) -> (x*y=w892:dbl)
        n171 = Add(x=w896, y=w892) -> (x+y=w894:dbl)
        "right wheels actual pwm" <- w894
        n172 = call <vilib>:"Set Duty Cycle and Frequency.vi"("Frequency [Hz]"=w915, "Duty Cycle"=w894, "PWM Ref In"=w926) -> ()  [unwired: 6 in, 2 out]
        n173 = call <vilib>:"Set Duty Cycle and Frequency.vi"("Frequency [Hz]"=w915, "Duty Cycle"=w894, "PWM Ref In"=w916) -> ()  [unwired: 6 in, 2 out]
        n174 = call <vilib>:"Set Duty Cycle and Frequency.vi"("Frequency [Hz]"=w915, "Duty Cycle"=w894, "PWM Ref In"=w917) -> ()  [unwired: 6 in, 2 out]
        "PID feedback Right" <- w922
      }
      n175 = while {
        stop <- FALSE stop-if-true
        # "(current-start)/(goal-start)"
        n176 = local read "state"() -> (w223:dbl)
        n177 = case shown="2" w223 {
          frame 0, Default {
            n178 = local write "scale"(0.0) -> ()
          }
          frame 2 {
            # "heading"
            # "distance to goal"
            n179 = local read "loc_theta"() -> (w232:dbl)
            n180 = local read "loc_y"() -> (w244:dbl)
            n181 = shared-variable "RT myRIO Target - Overlord\\Localization_Variables_r0.lvlib\\loc_x"() -> (w253:dbl)  [unwired: 1 in, 1 out]
            n182 = local read "start x 2"() -> (w249:dbl)
            n183 = Subtract(x=w249, y="x goal") -> (x-y=w252:dbl)
            n184 = Subtract(x="x goal", y=w249) -> (x-y=w248:dbl)
            n185 = Subtract(x=w253, y=w249) -> (x-y=w231:dbl)
            n186 = Sine(x=w232) -> (sin(x)=w238:dbl)
            n187 = Add(x=w231, y=w252) -> (x+y=w251:dbl)
            n188 = Multiply(x=w238, y=w231) -> (x*y=w239:dbl)
            n189 = local read "y goal"() -> (w241:dbl)
            n190 = Add(x=w239, y=w244) -> (x+y=w240:dbl)
            n191 = Divide(x=w251, y=w248) -> (x/y=w246:dbl)
            "percent away from x goal" <- w246
            n192 = Subtract(x=w240, y=w241) -> (x-y=w235:dbl)
            n193 = Greater?(x=w246, y=-0.25) -> (0:w247:bool)
            n194 = In Range and Coerce(upper limit="y goal upper limit mine", x=w235, lower limit="y goal lower limit mine") -> (coerced(x)=w236:dbl, In Range?=w237:bool)
            n195 = Sign(1:w246) -> (0:w245:dbl)
            n196 = case shown="True" w247 {
              tunnel: w246 -> [_ w268]
              tunnel: w245 -> [w263 w265]
              frame False {
                n197 = Multiply(x=1.0, y=w263) -> (x*y=→"scale":dbl)
              }
              frame True {
                n198 = Greater?(x=w268, y=0.0) -> (0:w266:bool)
                n199 = case shown="False" w266 {
                  tunnel: w265 -> [w271 _]
                  frame False {
                    n200 = Multiply(x=w271, y=0.85) -> (x*y=w269:dbl)
                    n201 = local write "scale"(w269) -> ()
                  }
                  frame True {
                    n202 = local write "scale"(0.0) -> ()
                    "goal reached" <- TRUE
                  }
                }
              }
            }
            n203 = Subtract(x=w235, y=w236) -> (x-y=w234:dbl)
            n204 = Sign(1:w234) -> (0:w233:dbl)
            n205 = case shown="True" w237 {
              tunnel: w233 -> [w255 _]
              frame False {
                n206 = case shown="-1, Default" w255 {
                  frame -1, Default {
                    n207 = local write "left setpoint"("left setpoint 3") -> ()
                    n208 = local write "right setpoint"("right setpoint 3") -> ()
                  }
                  frame 1 {
                    # "increase turn"
                    n209 = local write "right setpoint"("right setpoint 2") -> ()
                    n210 = local write "left setpoint"("left setpoint 2") -> ()
                  }
                }
              }
              frame True {
                n211 = local write "right setpoint"("right setpoint 7") -> ()
                n212 = local write "left setpoint"("left setpoint 7") -> ()
              }
            }
          }
          frame 3 {
            n213 = local write "scale"(0.0) -> ()
          }
          frame 4 {
            # "heading"
            # "distance to goal"
            n214 = local read "xstart_return"() -> (w291:dbl)
            n215 = shared-variable "RT myRIO Target - Overlord\\Localization_Variables_r0.lvlib\\loc_x"() -> (w292:dbl)  [unwired: 1 in, 1 out]
            n216 = local read "x goal"() -> (w293:dbl)
            n217 = local read "loc_theta"() -> (w278:dbl)
            n218 = Subtract(x=w292, y=w291) -> (x-y=w297:dbl)
            n219 = Subtract(x=w291, y=w293) -> (x-y=w277:dbl)
            n220 = local read "loc_y"() -> (w290:dbl)
            n221 = Add(x=w277, y=w297) -> (x+y=w296:dbl)
            n222 = Divide(x=w296, y=w277) -> (x/y=w276:dbl)
            "percent away from x goal 2" <- w276
            n223 = Multiply(x=w277, y=w276) -> (x*y=w275:dbl)
            n224 = Sine(x=w278) -> (sin(x)=w284:dbl)
            n225 = Less?(x=w276, y=0.25) -> (x < y?=w295:bool)
            n226 = Multiply(x=w284, y=w275) -> (x*y=w285:dbl)
            n227 = Sign(1:w276) -> (0:w294:dbl)
            n228 = case shown="True" w295 {
              tunnel: w276 -> [_ w312]
              tunnel: w294 -> [w307 w309]
              frame False {
                n229 = Multiply(x=1.0, y=w307) -> (x*y=w306:dbl)
                n230 = local write "scale"(w306) -> ()
              }
              frame True {
                n231 = Less?(x=w312, y=0.0) -> (x < y?=w310:bool)
                n232 = case shown="True" w310 {
                  tunnel: w309 -> [w315 _]
                  frame False {
                    n233 = Multiply(x=w315, y=0.85) -> (x*y=w313:dbl)
                    n234 = local write "scale"(w313) -> ()
                  }
                  frame True {
                    n235 = local write "scale"(0.0) -> ()
                    "goal reached 2" <- TRUE
                  }
                }
              }
            }
            n236 = Add(x=w285, y=w290) -> (x+y=w286:dbl)
            n237 = local read "y goal"() -> (w287:dbl)
            n238 = Subtract(x=w286, y=w287) -> (x-y=w281:dbl)
            n239 = In Range and Coerce(upper limit="y goal upper limit return", x=w281, lower limit="y goal lower limit return") -> (coerced(x)=w282:dbl, In Range?=w283:bool)
            n240 = Subtract(x=w281, y=w282) -> (x-y=w280:dbl)
            n241 = Sign(1:w280) -> (0:w279:dbl)
            n242 = case shown="False" w283 {
              tunnel: w279 -> [w299 _]
              frame False {
                n243 = case shown="-1, Default" w299 {
                  frame -1, Default {
                    n244 = local write "left setpoint"("left setpoint 4") -> ()
                    n245 = local write "right setpoint"("right setpoint 4") -> ()
                  }
                  frame 1 {
                    # "increase turn"
                    n246 = local write "left setpoint"("left setpoint 5") -> ()
                    n247 = local write "right setpoint"("right setpoint 5") -> ()
                  }
                }
              }
              frame True {
                n248 = local write "left setpoint"("left setpoint 6") -> ()
                n249 = local write "right setpoint"("right setpoint 6") -> ()
              }
            }
          }
          frame 5 {
            n250 = local write "scale"(0.0) -> ()
          }
        }
        n251 = local read "Encoder Reset"() -> (w229:bool)
        n252 = case shown="False" w229 {
          tunnel: [w319 w320] -> w228
          frame False {
            w319 = 1.0
            n253 = local write "reset x y 2"(w319) -> ()
          }
          frame True {
            w320 = 0.0
            n254 = local write "reset x y 2"(w320) -> ()
            "reset x y 2" <- w320
          }
        }
        "encoder stop switch" <- w228
        n255 = Not(x="motor killswitch") -> (.not. x?=w227:bool)
        n256 = Boolean To (0,1)(Boolean=w227) -> (0, 1=→"big red button":i16)
      }
      n257 = while {
        tunnel: w214 -> [w933]
        stop <- FALSE stop-if-true
        # "left mid"
        n258 = xnode "Read/Write Control"("FPGA VI Reference In"=w933) -> ("ENC.A_a.CNTR"=→"ENC.A_a.CNTR":u32, "ENC.A_b.CNTR"=→"ENC.A_b.CNTR":u32, "ENC.A_c.CNTR"=→"ENC.A_c.CNTR":u32, "ENC.B_a.CNTR"=→"ENC.B_a.CNTR":u32, "ENC.B_b.CNTR"=→"ENC.B_b.CNTR":u32, "ENC.B_c.CNTR"=→"ENC.B_c.CNTR":u32)  [unwired: 1 in, 2 out]
        n259 = xnode "Read/Write Control"("FPGA VI Reference In"=w933) -> ()  [unwired: 1 in, 3 out]
        n260 = Wait (ms)(milliseconds to wait=u32 20) -> ()  [unwired: 1 out]
        n261 = case shown="True" "Encoder Reset" {
          tunnel: w933 -> [_ w943]
          frame False {
          }
          frame True {
            n262 = flat-sequence {
              tunnel: w943 -> [w948]
              tunnel: [w946] -> w945
              tunnel: w945 -> [w950]
              tunnel: [w950] -> w944
              tunnel: w944 -> [w953]
              tunnel: [w952] -> _
              frame #0 {
                w947 = u8 60 ("SYS.SELECTA")
                w949 = u8 3 ("ENC.B_c.CNFG")
                n263 = xnode "Read/Write Control"("FPGA VI Reference In"=w948, "ENC.A_a.CNFG"=w949, "ENC.A_b.CNFG"=w949, "ENC.A_c.CNFG"=w949, "ENC.B_a.CNFG"=w949, "ENC.B_b.CNFG"=w949, "ENC.B_c.CNFG"=w949, "SYS.SELECTA"=w947, "SYS.SELECTB"=w947) -> ("FPGA VI Reference Out"=w946:refnum<k20>)  [unwired: 1 in, 1 out]
              }
              frame #1 {
                n264 = Wait (ms)(milliseconds to wait=u32 10) -> ()  [unwired: 1 out]
              }
              frame #2 {
                w954 = u8 1 ("ENC.B_c.CNFG")
                n265 = xnode "Read/Write Control"("FPGA VI Reference In"=w953, "ENC.A_a.CNFG"=w954, "ENC.A_b.CNFG"=w954, "ENC.A_c.CNFG"=w954, "ENC.B_a.CNFG"=w954, "ENC.B_b.CNFG"=w954, "ENC.B_c.CNFG"=w954) -> ("FPGA VI Reference Out"=w952:refnum<k20>)  [unwired: 1 in, 1 out]
              }
            }
          }
        }
      }
      n266 = while {
        stop <- w344 stop-if-true
        n267 = case shown="1" "state" {
          tunnel: [_ _ _ _ _ w751] -> w344
          frame 0, Default {
            (unwired) TRUE
            # "state 0=start"
            n268 = flat-sequence {
              frame #0 {
                n269 = local read "mining location"() -> (w348:dbl)
                n270 = case shown="-1" w348 {
                  tunnel: ["mining x 1" "mining x -1"] -> w345
                  tunnel: ["mining y 1" "mining y -1"] -> w347
                  tunnel: ["mining angle 1" "mining angle -1"] -> w346
                  frame 1, Default {
                  }
                  frame -1 {
                  }
                }
                "mining x" <- w345
                "mining y" <- w347
                "mining angle" <- w346
                "y goal" <- w347
                "angle goal" <- w346
                n271 = local write "x goal"(w345) -> ()
              }
              frame #1 {
                n272 = local read "state"() -> (w356:dbl)
                n273 = local write "stop motors"(0.0 ("stop motors")) -> ()
                n274 = Add(x=w356, y=1.0) -> (x+y=w358:dbl)
                n275 = local write "state"(w358) -> ()
              }
              frame #2 {
                n276 = disable-structure shown="Disabled" {
                  frame Disabled {
                    n277 = local read "state"() -> (w361:dbl)
                    n278 = Equal?(x=w361, y=1.0) -> (x = y?=w359:bool)
                    n279 = call "Display Message to User"("Enable"=w359) -> ()  [unwired: 9 in, 2 out]
                  }
                  frame Enabled {
                  }
                }
              }
            }
          }
          frame 1 {
            n280 = case shown="2" "start condition" {
              frame 1, Default {
                n281 = flat-sequence {
                  frame #0 {
                    n282 = call "Tick Count30"() -> ("Tick Count(mSec)"=w363:u32)
                    n283 = while {
                      shift-right: [w366] -> _
                      shift-left: w363 -> [w367]
                      shift-right: [w369] -> _
                      shift-left: 0 -> [w365]
                      stop <- w368 stop-if-true
                      # "left=right\ngoing down course pwm<0.5"
                      # "case 0 go straight"
                      n284 = call "Tick Count29"() -> ("Tick Count(mSec)"=w366:u32)
                      n285 = local write "right setpoint"("right 0") -> ()
                      n286 = Subtract(x=w366, y=w367) -> (x-y=w370:u32)
                      n287 = Add(x=w365, y=w370) -> (x+y=w369:u32)
                      n288 = local write "left setpoint"("left 0") -> ()
                      n289 = Greater Or Equal?(x=w369, y="t backward 7") -> (x >= y?=w368:bool)
                    }
                  }
                  frame #1 {
                    w375 = 0.0
                    n290 = local write "state"(2.0 ("state")) -> ()
                    n291 = local write "right setpoint"(w375) -> ()
                    n292 = local write "left setpoint"(w375) -> ()
                  }
                }
              }
              frame 2 {
                n293 = flat-sequence {
                  frame #0 {
                    # "if facing north | left side | > |right side|\nif facing south |left side | < |right side|"
                    n294 = call "Tick Count18"() -> ("Tick Count(mSec)"=w377:u32)
                    n295 = while {
                      shift-right: [w380] -> _
                      shift-left: 0 -> [w382]
                      shift-right: [w381] -> _
                      shift-left: w377 -> [w384]
                      stop <- w379 stop-if-true
                      # "one time turn"
                      n296 = call "Tick Count17"() -> ("Tick Count(mSec)"=w381:u32)
                      n297 = Subtract(x=w381, y=w384) -> (x-y=w383:u32)
                      n298 = local write "right setpoint"("right once") -> ()
                      n299 = Add(x=w382, y=w383) -> (x+y=w380:u32)
                      n300 = local write "left setpoint"("left once") -> ()
                      n301 = Greater Or Equal?(x=w380, y="t forward once") -> (x >= y?=w379:bool)
                    }
                  }
                  frame #1 {
                    w387 = 0.0
                    n302 = Wait (ms)(milliseconds to wait=u32 1000) -> ()  [unwired: 1 out]
                    n303 = local write "right setpoint"(w387) -> ()
                    n304 = local write "left setpoint"(w387) -> ()
                  }
                  frame #2 {
                    n305 = while {
                      i -> [w389]
                      stop <- FALSE stop-if-true
                      n306 = flat-sequence {
                        tunnel: w389 -> [w421]
                        frame #0 {
                          n307 = call "Tick Count3"() -> ("Tick Count(mSec)"=w391:u32)
                          n308 = while {
                            shift-right: [w395] -> _
                            shift-left: 0 -> [w397]
                            shift-right: [w396] -> _
                            shift-left: w391 -> [w399]
                            stop <- w394 stop-if-true
                            # "if facing north | left side | > |right side|\nif facing south |left side | < |right side|"
                            # "case 1 arc out"
                            n309 = call "Tick Count4"() -> ("Tick Count(mSec)"=w396:u32)
                            n310 = local write "right setpoint"("right 1") -> ()
                            n311 = Subtract(x=w396, y=w399) -> (x-y=w398:u32)
                            n312 = Add(x=w397, y=w398) -> (x+y=w395:u32)
                            n313 = local write "left setpoint"("left 1") -> ()
                            n314 = Greater Or Equal?(x=w395, y="t backward") -> (x >= y?=w394:bool)
                          }
                        }
                        frame #1 {
                          w403 = 0.0
                          n315 = Wait (ms)(milliseconds to wait=u32 1000) -> ()  [unwired: 1 out]
                          n316 = local write "right setpoint"(w403) -> ()
                          n317 = local write "left setpoint"(w403) -> ()
                        }
                        frame #2 {
                          n318 = call "Tick Count5"() -> ("Tick Count(mSec)"=w405:u32)
                          n319 = while {
                            shift-right: [w408] -> _
                            shift-left: 0 -> [w411]
                            shift-right: [w409] -> _
                            shift-left: w405 -> [w412]
                            stop <- w407 stop-if-true
                            # "if facing north | left side | > |right side|\nif facing south |left side | < |right side|"
                            # "case 1 arc out"
                            n320 = call "Tick Count6"() -> ("Tick Count(mSec)"=w409:u32)
                            n321 = local write "right setpoint"("right 2") -> ()
                            n322 = Subtract(x=w409, y=w412) -> (x-y=w410:u32)
                            n323 = Add(x=w411, y=w410) -> (x+y=w408:u32)
                            n324 = local write "left setpoint"("left 2") -> ()
                            n325 = Greater Or Equal?(x=w408, y="t forward") -> (x >= y?=w407:bool)
                          }
                        }
                        frame #3 {
                          w420 = 0.0
                          n326 = local write "right setpoint"(w420) -> ()
                          n327 = local write "left setpoint"(w420) -> ()
                          n328 = Add(x=1, y=w421) -> (x+y=w416:i32)
                          n329 = Quotient & Remainder(x=w416, y=4) -> (x-y*floor(x/y)=w418:i32)  [unwired: 1 out]
                          n330 = Equal To 0?(x=w418) -> (x = 0?=w417:bool)
                          n331 = case shown="True" w417 {
                            frame False {
                              n332 = Wait (ms)(milliseconds to wait=u32 1000) -> ()  [unwired: 1 out]
                            }
                            frame True {
                              n333 = call "Tick Count8"() -> ("Tick Count(mSec)"=w423:u32)
                              n334 = while {
                                shift-right: [w426] -> _
                                shift-left: 0 -> [w429]
                                shift-right: [w427] -> _
                                shift-left: w423 -> [w428]
                                stop <- w425 stop-if-true
                                # "do we have camera lock shared var"
                                n335 = shared-variable "RT myRIO Target - Overlord\\Localization_Variables_r0.lvlib\\Position_Lock"() -> (w432:bool)  [unwired: 1 in, 1 out]
                                n336 = case shown="False" w432 {
                                frame False {
                                }
                                frame True {
                                n337 = local write "state"(2.0) -> ()
                                }
                                }
                                n338 = call "Tick Count7"() -> ("Tick Count(mSec)"=w427:u32)
                                n339 = Subtract(x=w427, y=w428) -> (x-y=w431:u32)
                                n340 = Add(x=w429, y=w431) -> (x+y=w426:u32)
                                n341 = Greater Or Equal?(x=w426, y=u32 10000) -> (x >= y?=w425:bool)
                              }
                            }
                          }
                        }
                      }
                    }
                  }
                }
              }
              frame 3 {
                n342 = flat-sequence {
                  frame #0 {
                    # "one time turn"
                    # "if facing north | left side | > |right side|\nif facing south |left side | < |right side|"
                    n343 = call "Tick Count26"() -> ("Tick Count(mSec)"=w435:u32)
                    n344 = while {
                      shift-right: [w438] -> _
                      shift-left: 0 -> [w440]
                      shift-right: [w439] -> _
                      shift-left: w435 -> [w442]
                      stop <- w437 stop-if-true
                      n345 = call "Tick Count25"() -> ("Tick Count(mSec)"=w439:u32)
                      n346 = Subtract(x=w439, y=w442) -> (x-y=w441:u32)
                      n347 = local write "right setpoint"("right once 2") -> ()
                      n348 = local write "left setpoint"("left once 2") -> ()
                      n349 = Add(x=w440, y=w441) -> (x+y=w438:u32)
                      n350 = Greater Or Equal?(x=w438, y="t forward once 2") -> (x >= y?=w437:bool)
                    }
                  }
                  frame #1 {
                    w445 = 0.0
                    n351 = Wait (ms)(milliseconds to wait=u32 1000) -> ()  [unwired: 1 out]
                    n352 = local write "right setpoint"(w445) -> ()
                    n353 = local write "left setpoint"(w445) -> ()
                  }
                  frame #2 {
                    n354 = while {
                      i -> [w448]
                      stop <- w447 stop-if-true
                      (unwired) FALSE
                      n355 = flat-sequence {
                        tunnel: w448 -> [w480]
                        tunnel: [w473] -> w447
                        frame #0 {
                          n356 = call "Tick Count20"() -> ("Tick Count(mSec)"=w449:u32)
                          n357 = while {
                            shift-right: [w453] -> _
                            shift-left: 0 -> [w455]
                            shift-right: [w454] -> _
                            shift-left: w449 -> [w457]
                            stop <- w452 stop-if-true
                            # "if facing north | left side | > |right side|\nif facing south |left side | < |right side|"
                            # "case 1 arc out"
                            n358 = call "Tick Count19"() -> ("Tick Count(mSec)"=w454:u32)
                            n359 = Subtract(x=w454, y=w457) -> (x-y=w456:u32)
                            n360 = local write "right setpoint"("right 6") -> ()
                            n361 = Add(x=w455, y=w456) -> (x+y=w453:u32)
                            n362 = Greater Or Equal?(x=w453, y="t backward 2") -> (x >= y?=w452:bool)
                            n363 = local write "left setpoint"("left 6") -> ()
                          }
                        }
                        frame #1 {
                          w461 = 0.0
                          n364 = Wait (ms)(milliseconds to wait=u32 1000) -> ()  [unwired: 1 out]
                          n365 = local write "right setpoint"(w461) -> ()
                          n366 = local write "left setpoint"(w461) -> ()
                        }
                        frame #2 {
                          n367 = call "Tick Count22"() -> ("Tick Count(mSec)"=w463:u32)
                          n368 = while {
                            shift-right: [w466] -> _
                            shift-left: 0 -> [w469]
                            shift-right: [w467] -> _
                            shift-left: w463 -> [w470]
                            stop <- w465 stop-if-true
                            # "if facing north | left side | > |right side|\nif facing south |left side | < |right side|"
                            # "case 1 arc out"
                            n369 = call "Tick Count21"() -> ("Tick Count(mSec)"=w467:u32)
                            n370 = Subtract(x=w467, y=w470) -> (x-y=w468:u32)
                            n371 = local write "right setpoint"("right 7") -> ()
                            n372 = Add(x=w469, y=w468) -> (x+y=w466:u32)
                            n373 = Greater Or Equal?(x=w466, y="t forward 2") -> (x >= y?=w465:bool)
                            n374 = local write "left setpoint"("left 7") -> ()
                          }
                        }
                        frame #3 {
                          w479 = 0.0
                          n375 = local write "right setpoint"(w479) -> ()
                          n376 = local write "left setpoint"(w479) -> ()
                          n377 = Add(x=1, y=w480) -> (x+y=w475:i32)
                          n378 = Quotient & Remainder(x=w475, y=4) -> (x-y*floor(x/y)=w477:i32)  [unwired: 1 out]
                          n379 = Equal To 0?(x=w477) -> (x = 0?=w476:bool)
                          n380 = case shown="False" w476 {
                            selector: w476 -> [w481 _]
                            tunnel: [w481 w483] -> w473
                            frame False {
                              n381 = Wait (ms)(milliseconds to wait=u32 1000) -> ()  [unwired: 1 out]
                            }
                            frame True {
                              n382 = call "Tick Count24"() -> ("Tick Count(mSec)"=w484:u32)
                              n383 = while {
                                shift-right: [w488] -> _
                                shift-left: 0 -> [w491]
                                shift-right: [w489] -> _
                                shift-left: w484 -> [w490]
                                tunnel: [w486] -> w483
                                stop <- w487 stop-if-true
                                # "do we have camera lock shared var"
                                n384 = shared-variable "RT myRIO Target - Overlord\\Localization_Variables_r0.lvlib\\Position_Lock"() -> (w486:bool)  [unwired: 1 in, 1 out]
                                n385 = call "Tick Count23"() -> ("Tick Count(mSec)"=w489:u32)
                                n386 = Subtract(x=w489, y=w490) -> (x-y=w493:u32)
                                n387 = case shown="True" w486 {
                                frame False {
                                }
                                frame True {
                                n388 = local write "state"(2.0) -> ()
                                }
                                }
                                n389 = Add(x=w491, y=w493) -> (x+y=w488:u32)
                                n390 = Greater Or Equal?(x=w488, y=u32 10000) -> (x >= y?=w487:bool)
                              }
                            }
                          }
                        }
                      }
                    }
                  }
                }
              }
              frame 4 {
                n391 = while {
                  i -> [w495]
                  stop <- FALSE stop-if-true
                  n392 = flat-sequence {
                    tunnel: w495 -> [w508]
                    frame #0 {
                      n393 = call "Tick Count36"() -> ("Tick Count(mSec)"=w497:u32)
                      n394 = while {
                        shift-right: [w501] -> _
                        shift-left: 0 -> [w503]
                        shift-right: [w502] -> _
                        shift-left: w497 -> [w505]
                        stop <- w500 stop-if-true
                        # "if facing north | left side | > |right side|\nif facing south |left side | < |right side|"
                        # "case 1 arc out"
                        n395 = call "Tick Count35"() -> ("Tick Count(mSec)"=w502:u32)
                        n396 = local write "right setpoint"("right 10") -> ()
                        n397 = Subtract(x=w502, y=w505) -> (x-y=w504:u32)
                        n398 = Add(x=w503, y=w504) -> (x+y=w501:u32)
                        n399 = local write "left setpoint"("left 10") -> ()
                        n400 = Greater Or Equal?(x=w501, y="forward") -> (x >= y?=w500:bool)
                      }
                    }
                    frame #1 {
                      n401 = while {
                        tunnel: w508 -> [w510]
                        stop <- w509 stop-if-true
                        n402 = flat-sequence {
                          tunnel: w510 -> [w538]
                          tunnel: [w537] -> w509
                          frame #0 {
                            w511 = 0.0
                            n403 = Wait (ms)(milliseconds to wait=u32 1000) -> ()  [unwired: 1 out]
                            n404 = local write "right setpoint"(w511) -> ()
                            n405 = local write "left setpoint"(w511) -> ()
                          }
                          frame #1 {
                            n406 = call "Tick Count38"() -> ("Tick Count(mSec)"=w513:u32)
                            n407 = while {
                              shift-right: [w516] -> _
                              shift-left: 0 -> [w519]
                              shift-right: [w517] -> _
                              shift-left: w513 -> [w520]
                              stop <- w515 stop-if-true
                              # "if facing north | left side | > |right side|\nif facing south |left side | < |right side|"
                              # "case 1 arc out"
                              n408 = call "Tick Count37"() -> ("Tick Count(mSec)"=w517:u32)
                              n409 = Subtract(x=w517, y=w520) -> (x-y=w518:u32)
                              n410 = local write "right setpoint"("right 11") -> ()
                              n411 = Add(x=w519, y=w518) -> (x+y=w516:u32)
                              n412 = Greater Or Equal?(x=w516, y="timeforward") -> (x >= y?=w515:bool)
                              n413 = local write "left setpoint"("left 11") -> ()
                            }
                          }
                          frame #2 {
                            w524 = 0.0
                            n414 = Wait (ms)(milliseconds to wait=u32 1000) -> ()  [unwired: 1 out]
                            n415 = local write "right setpoint"(w524) -> ()
                            n416 = local write "left setpoint"(w524) -> ()
                          }
                          frame #3 {
                            n417 = call "Tick Count42"() -> ("Tick Count(mSec)"=w526:u32)
                            n418 = while {
                              shift-right: [w529] -> _
                              shift-left: 0 -> [w532]
                              shift-right: [w530] -> _
                              shift-left: w526 -> [w533]
                              stop <- w528 stop-if-true
                              # "if facing north | left side | > |right side|\nif facing south |left side | < |right side|"
                              # "case 1 arc out"
                              n419 = call "Tick Count41"() -> ("Tick Count(mSec)"=w530:u32)
                              n420 = local write "right setpoint"("right 12") -> ()
                              n421 = local write "left setpoint"("left 12") -> ()
                              n422 = Subtract(x=w530, y=w533) -> (x-y=w531:u32)
                              n423 = Add(x=w532, y=w531) -> (x+y=w529:u32)
                              n424 = Greater Or Equal?(x=w529, y="timeback") -> (x >= y?=w528:bool)
                            }
                          }
                          frame #4 {
                            w539 = 0.0
                            n425 = Add(x=1, y=w538) -> (x+y=w543:i32)
                            n426 = local write "right setpoint"(w539) -> ()
                            n427 = local write "left setpoint"(w539) -> ()
                            n428 = Quotient & Remainder(x=w543, y=4) -> (x-y*floor(x/y)=w541:i32)  [unwired: 1 out]
                            n429 = Equal To 0?(x=w541) -> (x = 0?=w542:bool)
                            n430 = case shown="True" w542 {
                              tunnel: [_ w546] -> w537
                              frame False {
                                n431 = Wait (ms)(milliseconds to wait=u32 1000) -> ()  [unwired: 1 out]
                              }
                              frame True {
                                n432 = call "Tick Count40"() -> ("Tick Count(mSec)"=w547:u32)
                                n433 = while {
                                shift-right: [w550] -> _
                                shift-left: 0 -> [w553]
                                shift-right: [w551] -> _
                                shift-left: w547 -> [w552]
                                tunnel: [w549] -> w546
                                stop <- w549 stop-if-true
                                # "do we have camera lock shared var"
                                n434 = shared-variable "RT myRIO Target - Overlord\\Localization_Variables_r0.lvlib\\Position_Lock"() -> (w556:bool)  [unwired: 1 in, 1 out]
                                n435 = case shown="True" w556 {
                                frame False {
                                }
                                frame True {
                                n436 = local write "state"(2.0) -> ()
                                }
                                }
                                n437 = call "Tick Count39"() -> ("Tick Count(mSec)"=w551:u32)
                                n438 = Subtract(x=w551, y=w552) -> (x-y=w555:u32)
                                n439 = Add(x=w553, y=w555) -> (x+y=w550:u32)
                                n440 = Greater Or Equal?(x=w550, y=u32 10000) -> (x >= y?=w549:bool)
                                }
                              }
                            }
                          }
                        }
                      }
                    }
                  }
                }
              }
              frame 5 {
                n441 = flat-sequence {
                  frame #0 {
                    n442 = while {
                      shift-right: [w562] -> _
                      shift-left: _ -> [w558]
                      shift-right: [w561] -> _
                      shift-left: _ -> [w559]
                      stop <- w560 stop-if-true
                      # "left=right\ngoing down course pwm<0.5"
                      # "case 0 go straight"
                      n443 = local write "right setpoint"("right 15") -> ()
                      n444 = local write "left setpoint"("left 15") -> ()
                      n445 = call "Tick Count31"() -> ("Tick Count(mSec)"=w561:u32)
                      n446 = Subtract(x=w561, y=w559) -> (x-y=w563:u32)
                      n447 = Add(x=w558, y=w563) -> (x+y=w562:u32)
                      n448 = Greater Or Equal?(x=w562, y="t backward 8") -> (x >= y?=w560:bool)
                    }
                  }
                  frame #1 {
                    w568 = 0.0
                    n449 = local write "state"(2.0 ("state")) -> ()
                    n450 = local write "right setpoint"(w568) -> ()
                    n451 = local write "left setpoint"(w568) -> ()
                  }
                }
              }
              frame 6 {
                n452 = flat-sequence {
                  frame #0 {
                    # "back up straight"
                    n453 = call "Tick Count10"() -> ("Tick Count(mSec)"=w569:u32)
                    n454 = while {
                      shift-right: [w573] -> _
                      shift-left: 0 -> [w575]
                      shift-right: [w574] -> _
                      shift-left: w569 -> [w577]
                      stop <- w571 stop-if-true
                      # "if facing north | left side | > |right side|\nif facing south |left side | < |right side|"
                      # "case 1 arc out"
                      n455 = call "Tick Count9"() -> ("Tick Count(mSec)"=w574:u32)
                      n456 = local write "right setpoint"("right 3") -> ()
                      n457 = Subtract(x=w574, y=w577) -> (x-y=w576:u32)
                      n458 = Add(x=w575, y=w576) -> (x+y=w573:u32)
                      n459 = local write "left setpoint"("left 3") -> ()
                      n460 = Greater Or Equal?(x=w573, y="onetime 6") -> (x >= y?=w571:bool)
                    }
                  }
                  frame #1 {
                    n461 = while {
                      i -> [w580]
                      stop <- w581 stop-if-true
                      n462 = flat-sequence {
                        tunnel: w580 -> [w609]
                        tunnel: [w608] -> w581
                        frame #0 {
                          w582 = 0.0
                          n463 = Wait (ms)(milliseconds to wait=u32 1000) -> ()  [unwired: 1 out]
                          n464 = local write "right setpoint"(w582) -> ()
                          n465 = local write "left setpoint"(w582) -> ()
                        }
                        frame #1 {
                          n466 = call "Tick Count12"() -> ("Tick Count(mSec)"=w584:u32)
                          n467 = while {
                            shift-right: [w587] -> _
                            shift-left: 0 -> [w590]
                            shift-right: [w588] -> _
                            shift-left: w584 -> [w591]
                            stop <- w586 stop-if-true
                            # "if facing north | left side | > |right side|\nif facing south |left side | < |right side|"
                            # "case 1 arc out"
                            n468 = call "Tick Count11"() -> ("Tick Count(mSec)"=w588:u32)
                            n469 = local write "right setpoint"("right 4") -> ()
                            n470 = Subtract(x=w588, y=w591) -> (x-y=w589:u32)
                            n471 = Add(x=w590, y=w589) -> (x+y=w587:u32)
                            n472 = Greater Or Equal?(x=w587, y="backward 6") -> (x >= y?=w586:bool)
                            n473 = local write "left setpoint"("left 4") -> ()
                          }
                        }
                        frame #2 {
                          w595 = 0.0
                          n474 = Wait (ms)(milliseconds to wait=u32 1000) -> ()  [unwired: 1 out]
                          n475 = local write "right setpoint"(w595) -> ()
                          n476 = local write "left setpoint"(w595) -> ()
                        }
                        frame #3 {
                          n477 = call "Tick Count16"() -> ("Tick Count(mSec)"=w597:u32)
                          n478 = while {
                            shift-right: [w600] -> _
                            shift-left: 0 -> [w603]
                            shift-right: [w601] -> _
                            shift-left: w597 -> [w604]
                            stop <- w599 stop-if-true
                            # "if facing north | left side | > |right side|\nif facing south |left side | < |right side|"
                            # "case 1 arc out"
                            n479 = call "Tick Count15"() -> ("Tick Count(mSec)"=w601:u32)
                            n480 = local write "right setpoint"("right 5") -> ()
                            n481 = local write "left setpoint"("left 5") -> ()
                            n482 = Subtract(x=w601, y=w604) -> (x-y=w602:u32)
                            n483 = Add(x=w603, y=w602) -> (x+y=w600:u32)
                            n484 = Greater Or Equal?(x=w600, y="forward 6") -> (x >= y?=w599:bool)
                          }
                        }
                        frame #4 {
                          w610 = 0.0
                          n485 = local write "right setpoint"(w610) -> ()
                          n486 = local write "left setpoint"(w610) -> ()
                          n487 = Add(x=1, y=w609) -> (x+y=w614:i32)
                          n488 = Quotient & Remainder(x=w614, y=4) -> (x-y*floor(x/y)=w612:i32)  [unwired: 1 out]
                          n489 = Equal To 0?(x=w612) -> (x = 0?=w613:bool)
                          n490 = case shown="True" w613 {
                            tunnel: [_ w617] -> w608
                            frame False {
                              n491 = Wait (ms)(milliseconds to wait=u32 1000) -> ()  [unwired: 1 out]
                            }
                            frame True {
                              n492 = call "Tick Count14"() -> ("Tick Count(mSec)"=w618:u32)
                              n493 = while {
                                shift-right: [w621] -> _
                                shift-left: 0 -> [w624]
                                shift-right: [w622] -> _
                                shift-left: w618 -> [w623]
                                tunnel: [w620] -> w617
                                stop <- w620 stop-if-true
                                # "do we have camera lock shared var"
                                n494 = shared-variable "RT myRIO Target - Overlord\\Localization_Variables_r0.lvlib\\Position_Lock"() -> (w627:bool)  [unwired: 1 in, 1 out]
                                n495 = case shown="True" w627 {
                                frame False {
                                }
                                frame True {
                                n496 = local write "state"(2.0) -> ()
                                }
                                }
                                n497 = call "Tick Count13"() -> ("Tick Count(mSec)"=w622:u32)
                                n498 = Subtract(x=w622, y=w623) -> (x-y=w626:u32)
                                n499 = Add(x=w624, y=w626) -> (x+y=w621:u32)
                                n500 = Greater Or Equal?(x=w621, y=u32 10000) -> (x >= y?=w620:bool)
                              }
                            }
                          }
                        }
                      }
                    }
                  }
                }
              }
              frame 7 {
                n501 = flat-sequence {
                  frame #0 {
                    # "if facing north | left side | > |right side|\nif facing south |left side | < |right side|"
                    n502 = call "Tick Count50"() -> ("Tick Count(mSec)"=w630:u32)
                    n503 = while {
                      shift-right: [w633] -> _
                      shift-left: 0 -> [w635]
                      shift-right: [w634] -> _
                      shift-left: w630 -> [w637]
                      stop <- w632 stop-if-true
                      # "one time turn"
                      n504 = call "Tick Count49"() -> ("Tick Count(mSec)"=w634:u32)
                      n505 = Subtract(x=w634, y=w637) -> (x-y=w636:u32)
                      n506 = local write "right setpoint"("right once 5") -> ()
                      n507 = Add(x=w635, y=w636) -> (x+y=w633:u32)
                      n508 = local write "left setpoint"("left once 5") -> ()
                      n509 = Greater Or Equal?(x=w633, y="t forward once 5") -> (x >= y?=w632:bool)
                    }
                  }
                  frame #1 {
                    w640 = 0.0
                    n510 = Wait (ms)(milliseconds to wait=u32 1000) -> ()  [unwired: 1 out]
                    n511 = local write "right setpoint"(w640) -> ()
                    n512 = local write "left setpoint"(w640) -> ()
                  }
                  frame #2 {
                    n513 = while {
                      i -> [w642]
                      stop <- FALSE stop-if-true
                      n514 = flat-sequence {
                        tunnel: w642 -> [w674]
                        frame #0 {
                          n515 = call "Tick Count44"() -> ("Tick Count(mSec)"=w644:u32)
                          n516 = while {
                            shift-right: [w648] -> _
                            shift-left: 0 -> [w650]
                            shift-right: [w649] -> _
                            shift-left: w644 -> [w652]
                            stop <- w647 stop-if-true
                            # "if facing north | left side | > |right side|\nif facing south |left side | < |right side|"
                            # "case 1 arc out"
                            n517 = call "Tick Count43"() -> ("Tick Count(mSec)"=w649:u32)
                            n518 = local write "right setpoint"("right 16") -> ()
                            n519 = Subtract(x=w649, y=w652) -> (x-y=w651:u32)
                            n520 = Add(x=w650, y=w651) -> (x+y=w648:u32)
                            n521 = local write "left setpoint"("left 16") -> ()
                            n522 = Greater Or Equal?(x=w648, y="t backward 5") -> (x >= y?=w647:bool)
                          }
                        }
                        frame #1 {
                          w656 = 0.0
                          n523 = Wait (ms)(milliseconds to wait=u32 1000) -> ()  [unwired: 1 out]
                          n524 = local write "right setpoint"(w656) -> ()
                          n525 = local write "left setpoint"(w656) -> ()
                        }
                        frame #2 {
                          n526 = call "Tick Count46"() -> ("Tick Count(mSec)"=w658:u32)
                          n527 = while {
                            shift-right: [w661] -> _
                            shift-left: 0 -> [w664]
                            shift-right: [w662] -> _
                            shift-left: w658 -> [w665]
                            stop <- w660 stop-if-true
                            # "if facing north | left side | > |right side|\nif facing south |left side | < |right side|"
                            # "case 1 arc out"
                            n528 = call "Tick Count45"() -> ("Tick Count(mSec)"=w662:u32)
                            n529 = local write "right setpoint"("right 17") -> ()
                            n530 = Subtract(x=w662, y=w665) -> (x-y=w663:u32)
                            n531 = Add(x=w664, y=w663) -> (x+y=w661:u32)
                            n532 = local write "left setpoint"("left 17") -> ()
                            n533 = Greater Or Equal?(x=w661, y="t forward 5") -> (x >= y?=w660:bool)
                          }
                        }
                        frame #3 {
                          w673 = 0.0
                          n534 = local write "right setpoint"(w673) -> ()
                          n535 = local write "left setpoint"(w673) -> ()
                          n536 = Add(x=1, y=w674) -> (x+y=w669:i32)
                          n537 = Quotient & Remainder(x=w669, y=4) -> (x-y*floor(x/y)=w671:i32)  [unwired: 1 out]
                          n538 = Equal To 0?(x=w671) -> (x = 0?=w670:bool)
                          n539 = case shown="True" w670 {
                            frame False {
                              n540 = Wait (ms)(milliseconds to wait=u32 1000) -> ()  [unwired: 1 out]
                            }
                            frame True {
                              n541 = call "Tick Count48"() -> ("Tick Count(mSec)"=w676:u32)
                              n542 = while {
                                shift-right: [w679] -> _
                                shift-left: 0 -> [w682]
                                shift-right: [w680] -> _
                                shift-left: w676 -> [w681]
                                stop <- w678 stop-if-true
                                # "do we have camera lock shared var"
                                n543 = shared-variable "RT myRIO Target - Overlord\\Localization_Variables_r0.lvlib\\Position_Lock"() -> (w685:bool)  [unwired: 1 in, 1 out]
                                n544 = case shown="True" w685 {
                                frame False {
                                }
                                frame True {
                                n545 = local write "state"(2.0) -> ()
                                }
                                }
                                n546 = call "Tick Count47"() -> ("Tick Count(mSec)"=w680:u32)
                                n547 = Subtract(x=w680, y=w681) -> (x-y=w684:u32)
                                n548 = Add(x=w682, y=w684) -> (x+y=w679:u32)
                                n549 = Greater Or Equal?(x=w679, y=u32 10000) -> (x >= y?=w678:bool)
                              }
                            }
                          }
                        }
                      }
                    }
                  }
                }
              }
              frame 8 {
                n550 = local write "state"(2.0) -> ()
              }
            }
          }
          frame 2 {
            # "state 1=forward"
            n551 = while {
              stop <- w688 stop-if-true
              (unwired) FALSE
              n552 = flat-sequence {
                tunnel: [w697] -> w688
                frame #0 {
                  n553 = local write "stop motors"(1.0) -> ()
                }
                frame #1 {
                  n554 = while {
                    stop <- w692 stop-if-true
                    n555 = local read "x goal"() -> (w691:dbl)
                    n556 = local read "loc_x"() -> (w690:dbl)
                    n557 = Greater Or Equal?(x=w690, y=w691) -> (x >= y?=w692:bool)
                  }
                }
                frame #2 {
                  n558 = local read "state"() -> (w693:dbl)
                  n559 = local write "stop motors"(0.0) -> ()
                  n560 = Add(x=w693, y=1.0) -> (x+y=w695:dbl)
                  n561 = local write "state"(w695) -> ()
                }
                frame #3 {
                  n562 = disable-structure shown="Enabled" {
                    disable-tunnel: [w698 TRUE] -> w697
                    frame Disabled {
                      n563 = local read "state"() -> (w701:dbl)
                      n564 = Equal?(x=w701, y=3.0) -> (x = y?=w699:bool)
                      n565 = call "Display Message to User2"("Enable"=w699) -> ("OK"=w698:bool)  [unwired: 9 in, 1 out]
                    }
                    frame Enabled {
                    }
                  }
                }
              }
            }
          }
          frame 3 {
            # "state 2=dig"
            n566 = while {
              stop <- w703 stop-if-true
              (unwired) FALSE
              n567 = flat-sequence {
                tunnel: [w715] -> w703
                frame #0 {
                  n568 = disable-structure shown="Disabled" {
                    frame Disabled {
                      n569 = while {
                        stop <- w706 stop-if-true
                        n570 = shared-variable "RT myRIO Target - Overlord\\Mining_Variables_r0.lvlib\\Mine or Dump"(i16 1 ("Mine or Dump")) -> ()  [unwired: 1 in, 1 out]
                        n571 = shared-variable "RT myRIO Target - Overlord\\Mining_Variables_r0.lvlib\\Mining Complete"() -> (w705:bool)  [unwired: 1 in, 1 out]
                        n572 = Or(x=w705, y="digging complete?") -> (x .or. y?=w706:bool)
                      }
                    }
                    frame Enabled {
                    }
                  }
                }
                frame #1 {
                  n573 = local read "state"() -> (w713:dbl)
                  n574 = local write "angle goal"(0.0) -> ()
                  n575 = Wait (ms)(milliseconds to wait=u32 5000) -> ()  [unwired: 1 out]
                  n576 = local write "y goal"("dump y") -> ()
                  n577 = local write "x goal"("dump x") -> ()
                  n578 = Add(x=w713, y=1.0) -> (x+y=w712:dbl)
                  n579 = local write "state"(w712) -> ()
                }
                frame #2 {
                  n580 = disable-structure shown="Enabled" {
                    disable-tunnel: [w716 TRUE] -> w715
                    frame Disabled {
                      n581 = local read "state"() -> (w719:dbl)
                      n582 = Equal?(x=w719, y=4.0) -> (x = y?=w717:bool)
                      n583 = call "Display Message to User8"("Enable"=w717) -> ("OK"=w716:bool)  [unwired: 9 in, 1 out]
                    }
                    frame Enabled {
                    }
                  }
                }
              }
            }
          }
          frame 4 {
            # "state 3=return"
            n584 = while {
              stop <- w721 stop-if-true
              (unwired) FALSE
              # "dialog for testing and move to next case"
              # "measurement and control"
              # "chill and make sure loc is good"
              # "house keeping variables"
              n585 = flat-sequence {
                tunnel: [w745] -> w721
                frame #0 {
                  n586 = local write "stop motors"(1.0) -> ()
                  n587 = local read "right setpoint"() -> (w722:dbl)
                  n588 = local read "left setpoint"() -> (w723:dbl)
                  n589 = local write "left setpoint"(w722) -> ()
                  n590 = local write "right setpoint"(w723) -> ()
                }
                frame #1 {
                  n591 = call "Tick Count33"() -> ("Tick Count(mSec)"=w725:u32)
                  n592 = while {
                    shift-right: [w732] -> _
                    shift-left: w725 -> [w731]
                    shift-right: [w730] -> _
                    shift-left: 0 -> [w733]
                    stop <- w737 stop-if-true
                    n593 = call "Tick Count32"() -> ("Tick Count(mSec)"=w732:u32)
                    n594 = Subtract(x=w732, y=w731) -> (x-y=w734:u32)
                    n595 = local read "x goal"() -> (w736:dbl)
                    n596 = local read "loc_x"() -> (w735:dbl)
                    n597 = Add(x=w733, y=w734) -> (x+y=w730:u32)
                    n598 = Less Or Equal?(x=w735, y=w736) -> (x <= y?=w737:bool)
                    n599 = Quotient & Remainder(x=w730, y="timer control") -> (x-y*floor(x/y)=w728:u32)  [unwired: 1 out]
                    n600 = Equal To 0?(x=w728) -> (x = 0?=w727:bool)
                    n601 = case shown="True" w727 {
                      frame False {
                      }
                      frame True {
                        n602 = flat-sequence {
                          frame #0 {
                            n603 = local write "stop motors"(0.0) -> ()
                          }
                          frame #1 {
                            n604 = Wait (ms)(milliseconds to wait=u32 1000) -> ()  [unwired: 1 out]
                          }
                          frame #2 {
                            n605 = local write "stop motors"(1.0) -> ()
                          }
                        }
                      }
                    }
                  }
                }
                frame #2 {
                  n606 = local read "state"() -> (w742:dbl)
                  n607 = local write "stop motors"(0.0) -> ()
                  n608 = Add(x=w742, y=1.0) -> (x+y=w744:dbl)
                  n609 = local write "state"(w744) -> ()
                }
                frame #3 {
                  n610 = disable-structure shown="Enabled" {
                    disable-tunnel: [w746 TRUE] -> w745
                    frame Disabled {
                      n611 = local read "state"() -> (w749:dbl)
                      n612 = Equal?(x=w749, y=5.0) -> (x = y?=w747:bool)
                      n613 = call "Display Message to User5"("Enable"=w747) -> ("OK"=w746:bool)  [unwired: 9 in, 1 out]
                    }
                    frame Enabled {
                    }
                  }
                }
              }
            }
          }
          frame 5 {
            # "state 4=dump"
            n614 = flat-sequence {
              tunnel: [w762] -> w751
              frame #0 {
                n615 = disable-structure shown="Disabled" {
                  frame Disabled {
                    n616 = while {
                      stop <- w754 stop-if-true
                      n617 = shared-variable "RT myRIO Target - Overlord\\Mining_Variables_r0.lvlib\\Mine or Dump"(i16 -1 ("Mine or Dump")) -> ()  [unwired: 1 in, 1 out]
                      n618 = shared-variable "RT myRIO Target - Overlord\\Mining_Variables_r0.lvlib\\Dumping Complete"() -> (w753:bool)  [unwired: 1 in, 1 out]
                      n619 = Or(x=w753, y="dumping complete") -> (x .or. y?=w754:bool)
                    }
                  }
                  frame Enabled {
                  }
                }
              }
              frame #1 {
                n620 = local write "start condition"(8.0) -> ()
                n621 = local write "state"(0.0) -> ()
                n622 = local read "mining location"() -> (w760:dbl)
                n623 = Wait (ms)(milliseconds to wait=u32 5000) -> ()  [unwired: 1 out]
                n624 = Multiply(x=w760, y=-1.0) -> (x*y=w759:dbl)
                n625 = local write "mining location"(w759) -> ()
              }
              frame #2 {
                n626 = disable-structure shown="Enabled" {
                  disable-tunnel: [w763 TRUE] -> w762
                  frame Disabled {
                    n627 = local read "state"() -> (w766:dbl)
                    n628 = Equal?(x=w766, y=0.0) -> (x = y?=w764:bool)
                    n629 = call "Display Message to User9"("Enable"=w764) -> ("OK"=w763:bool)  [unwired: 9 in, 1 out]
                  }
                  frame Enabled {
                  }
                }
              }
            }
          }
        }
      }
      n630 = while {
        shift-right: [w218] -> _
        shift-left: 0 -> [w220]
        shift-right: [w219] -> _
        shift-left: w205 -> [w222]
        stop <- w217 stop-if-true
        n631 = call "Tick Count27"() -> ("Tick Count(mSec)"=w219:u32)
        n632 = Subtract(x=w219, y=w222) -> (x-y=w221:u32)
        n633 = Add(x=w220, y=w221) -> (x+y=w218:u32)
        n634 = Greater Or Equal?(x=w218, y="t backward 6") -> (x >= y?=w217:bool)
      }
      n635 = call "Tick Count"() -> ("Tick Count(uSec)"=w215:u32)
      n636 = while {
        shift-right: [w972] -> _
        shift-left: _ -> [w971]
        shift-right: [w969] -> _
        shift-left: w215 -> [w968]
        tunnel: w213 -> [w979]
        stop <- FALSE stop-if-true
        n637 = xnode "Read/Write Control"("FPGA VI Reference In"=w979) -> ("ENC.A_a.CNTR"=w978:u32, "ENC.A_b.CNTR"=w977:u32, "ENC.A_c.CNTR"=w976:u32, "ENC.B_a.CNTR"=w975:u32, "ENC.B_b.CNTR"=w974:u32, "ENC.B_c.CNTR"=w973:u32)  [unwired: 1 in, 2 out]
        n638 = call "Wait"("Count(mSec)"=u32 20) -> ()  [unwired: 1 out]
        n639 = Build Array(w978, w977, w976, w975, w974, w973) -> (w972:u32[])
        n640 = Subtract(x=w972, y=w971) -> (x-y=w970:u32[])
        n641 = call "Tick Count2"() -> ("Tick Count(uSec)"=w969:u32)
        n642 = Index Array(array=w970) -> (element #1=w967:u32, element #2=w966:u32, element #3=w965:u32, element #4=w964:u32, element #5=w963:u32, element #6=w962:u32)  [unwired: 6 in]
        n643 = Subtract(x=w969, y=w968) -> (x-y=w961:u32)
        n644 = call "Encoder-Velocity_Conversion (SubVI).vi"("delta  Encoder Count"=w967, "dt (uSec)"=w961) -> ("Rotational Velocity (RPS)"=w958:dbl)  [unwired: 7 in, 2 out]
        "LR Rot Velocity (rot/s)" <- w958
        n645 = call "Encoder-Velocity_Conversion (SubVI).vi"("delta  Encoder Count"=w964, "dt (uSec)"=w961) -> ("Rotational Velocity (RPS)"=w955:dbl)  [unwired: 7 in, 2 out]
        "RR Rot Velocity (rot/s)" <- w955
        n646 = call "Encoder-Velocity_Conversion (SubVI).vi"("delta  Encoder Count"=w963, "dt (uSec)"=w961) -> ("Rotational Velocity (RPS)"=w959:dbl)  [unwired: 7 in, 2 out]
        "RM Linear Velocity (rot/s)" <- w959
        n647 = call "Encoder-Velocity_Conversion (SubVI).vi"("delta  Encoder Count"=w962, "dt (uSec)"=w961) -> ("Rotational Velocity (RPS)"=w960:dbl)  [unwired: 7 in, 2 out]
        "RF Linear Velocity (rot/s)" <- w960
        n648 = call "Encoder-Velocity_Conversion (SubVI).vi"("delta  Encoder Count"=w966, "dt (uSec)"=w961) -> ("Rotational Velocity (RPS)"=w957:dbl)  [unwired: 7 in, 2 out]
        "LM Rot Velocity (rot/s)" <- w957
        n649 = call "Encoder-Velocity_Conversion (SubVI).vi"("delta  Encoder Count"=w965, "dt (uSec)"=w961) -> ("Rotational Velocity (RPS)"=w956:dbl)  [unwired: 7 in, 2 out]
        "LF Rot Velocity (rot/s)" <- w956
        n650 = Bundle("Rotational Velocity (RPS)"=w958, "Rotational Velocity (RPS)"=w957, "Rotational Velocity (RPS)"=w956, "Rotational Velocity (RPS)"=w955, "Rotational Velocity (RPS)"=w959, "Rotational Velocity (RPS)"=w960) -> ()  [unwired: 1 in, 1 out]
      }
    }
  }
